vi "AlliGator Decay Fit Parameter Map Actions.vi"(0 "AlliGator Q Elements in":T6[](array[typedef]), 1 "VI in":refnum<vi>, 2 "Script in":bool, 5 "data value reference":refnum<data-value>, 7 "AlliGator Q Event in":T7=enum."GUI:Idle", 9 "Data":variant, 11 "error in (no error)":errorcluster, 12 "AlliGator Ctrl Refnums":T8) -> (3 "Script out":bool, 4 "AlliGator Q Elements out":T6[](array[typedef]), 6 "Data Value Reference out":refnum<data-value>, 10 "[Notebook Message]":T1[](array[typedef]) {"Message Style"."Font Size" min=6.0 step=1.0}, 15 "error out":errorcluster)   [LabVIEW 2021, in "AlliGator Decay Fit Parameter Map.lvlib"]
doc: "Processes AlliGator decay fit parameter map-related actions."
uses:
  AlliGator/Decay Fit Parameter Map/AlliGator Decay Fit Parameter Map.lvlib
  AlliGator/Internal Variables/AlliGator Internal Variables v2.ctl
  <vilib>/vision/Image Controls.llb/IMAQ Image.ctl
  AlliGator/Internal Variables/AlliGator Gate Image Set.ctl
  AlliGator/Files/AlliGator FLI Dataset Type.ctl
  AlliGator/Files/AlliGator Data Series Type.ctl
  AlliGator/Dual-Channel Datasets/AlliGator Dataset Channel.ctl
  AlliGator/Settings/AlliGator Gate Arithmetic.ctl
  AlliGator/Source Image/AlliGator Displayed Image.ctl
  Image/Named ROI Description.ctl
  AlliGator/Phasor Graph/AlliGator Decay Metadata v3.ctl
  AlliGator/Decay Analysis/Decay Preprocessing/AlliGator Decay Background Subtraction Info.ctl
  AlliGator/Decay Analysis/Decay Preprocessing/AlliGator Baseline Subtraction Method.ctl
  Graphs/XY Graph/XY Graph Plot Shift Parameters.ctl
  Graphs/XY Graph/XY Graph Plot Shift Method.ctl
  AlliGator/Decay Analysis/Decay Preprocessing/AlliGator Decay Extrapolation Parameters.ctl
  Phasor/Calibration Phasor (m, phi).ctl
  Phasor/Phasor Reference Series.ctl
  Phasor/Phasor Calibration Map v2.ctl
  Phasor/Phasor (g, s).ctl
  AlliGator/Phasor Graph/AlliGator Raw Phasor Plot Data v5.ctl
  Phasor/Phasor Standard Deviation Options.ctl
  AlliGator/Phasor Plot/AlliGator Phasor Multi-Harmonic Data.ctl
  Phasor/Phasor Harmonic Data.ctl
  AlliGator/Decay Fit Parameter Map/AlliGator Decay Fit Options & Parameters v4.ctl
  Fits/IRF(X)PSED/Decay Fit Options v4.ctl
  Fits/Decay Convolution/Decay Model.ctl
  Fits/Residual Type.ctl
  Fits/IRF(X)PSED/Fit Weights Type v2.ctl
  Fits/Non-linear Fitting Method v2.ctl
  Fits/Fit Calculation Method.ctl
  Fits/Non-linear Fitting Algorithm.ctl
  AlliGator/Decay Analysis/Decay Fit/AlliGator Decay Fit Parameter Constraints 2.ctl
  Fits/IRF(X)PSED/Decay Fit Parameters In List.ctl
  Fits/IRF(X)PSED/MLE Baseline Offset Type.ctl
  AlliGator/Decay Analysis/Decay Preprocessing/AlliGator Decay Preprocessing Parameters.ctl
  Fits/IRF(X)PSED/Decay Fit Parameters & Derived Quantities List v2.ctl
  Fits/IRF(X)PSED/Decay Fit Result Constraint.ctl
  AlliGator/Decay Fit Parameter Map/AlliGator Parameter Maps Data.ctl
  AlliGator/Action Engine/AlliGator Q Event.ctl
  AlliGator/GUI/AlliGator Ctrl Refnums.ctl
  AlliGator/GUI/AlliGator Other Ctrl Refnums.ctl
  AlliGator/GUI/AlliGator State Indicator.ctl
  AlliGator/GUI/AlliGator Main Window Tabs.ctl
  AlliGator/GUI/AlliGator Phasor Plot Ctrl Refnums.ctl
  AlliGator/GUI/AlliGator Phasor Graph Ctrl Refnums.ctl
  Phasor/Phasor Calibration Type.ctl
  AlliGator/GUI/AlliGator Dataset Ctrl Refnums.ctl
  AlliGator/GUI/AlliGator Registered Events Ctrl Refnums.ctl
  AlliGator/GUI/AlliGator Image Histogram Control Refnums.ctl
  Histograms/Linear Histogram Options.ctl
  Histograms/Histogram Bin Option.ctl
  Histograms/Histogram Bin Position.ctl
  AlliGator/Decay Fit Parameter Map/AlliGator Decay Fit Map Control Refnums.ctl
  AlliGator/Parameter Map/AlliGator Parameter Map Control Refnums.ctl
  AlliGator/Action Engine/AlliGator Q Element.ctl
  Notebook/Notebook Message Object.ctl
  Rich Text Box/Text Formatting.ctl
  Rich Text Box/Text Colors.ctl
  Rich Text Box/Text Style.ctl
  Rich Text Box/Text Alignment.ctl
  AlliGator/Action Engine/Alligator Elements Order in Action Stack.ctl
  AlliGator/Globals, Variables, Constants/AlliGator Variables List.ctl
  AlliGator/GUI/AlliGator Image Display Type.ctl
  Palette/Image Palette Information.ctl
  Image/Image Display Palette Type.ctl
  Files/Load-Save File Info.ctl
  Rich Text Box/Text Format List.ctl
  AlliGator/GUI/AlliGator Image Mouse Up Event Data.ctl
  Image/Image ROI Descriptor.ctl
  Image/Image Contour Definition.ctl
  Image/Image Contour ID.ctl
  Image/Image ROI Type.ctl
  Image/Image Control Refnum.ctl
  AlliGator/Decay Fit Parameter Map/AlliGator Decay Parameter Map Update Event Data.ctl
  AlliGator/GUI/AlliGator Windows List.ctl
  c5217346-0728-4db9-a30e-52dae72b7cfc.vi
  Variant/Variant to Data/Variant to Boolean.vi
  AlliGator/Action Engine/AlliGator Add Single Action to Stack.vi
  Variant/Variant to Data/Variant to [String].vi
  Variant/Variant to Data/Variant to String.vi
  Variant/Variant to Data/Variant to I32.vi
  AlliGator/Local Decay Window/AlliGator Local Decay Window.lvlib
  Fits/Fits.lvlib
  AlliGator/Action Engine/AlliGator Action Engine.lvlib
  GUI/GUI.lvlib
  Variant/Variant to Data/Variant to Data.lvlib
  AlliGator/Globals, Variables, Constants/AlliGator Globals, Variables & Constants.lvlib
  Palette/Palette.lvlib
  AlliGator/GUI/AlliGator GUI.lvlib
  Image/Image.lvlib
  Files/Files.lvlib
  Sound/Sound.lvlib
  AlliGator/Parameter Map/AlliGator Parameter Map.lvlib
  Utilities/Utilities.lvlib
  Notebook/Notebook.lvlib
  Phasor/Phasor.lvlib
  AlliGator/Decay Analysis/Decay Preprocessing/AlliGator Decay Preprocessing.lvlib
  Graphs/XY Graph/XY Graph Add-Ons.lvlib
  AlliGator/Phasor Graph/AlliGator Phasor Graph.lvlib
  AlliGator/Files/AlliGator Files.lvlib
  AlliGator/Internal Variables/AlliGator Internal Variables.lvlib
  AlliGator/Phasor Plot/AlliGator Phasor Plot.lvlib
  AlliGator/Source Image/AlliGator Source Image.lvlib
  AlliGator/Decay Analysis/Decay Fit/AlliGator Decay Fit.lvlib
  AlliGator/Settings/AlliGator Settings.lvlib
  Rich Text Box/Rich Text Box.lvlib
  AlliGator/Dual-Channel Datasets/AlliGator Dual-Channel Datasets.lvlib
  Histograms/Histogram Window.lvlib
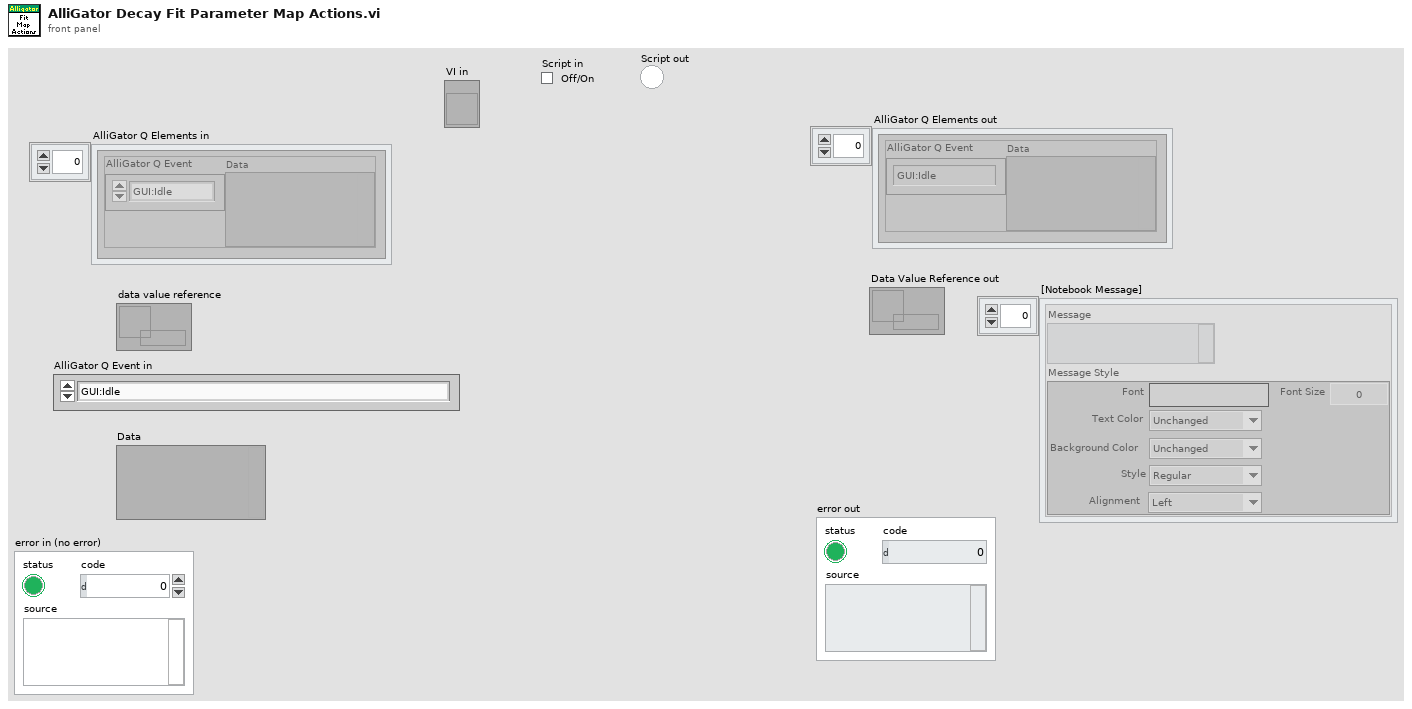
[diagram p1: front panel]
types:
  T1 = typedef "Notebook.lvlib/Notebook Message Object.ctl" = cluster{"Message":string, "Message Style":T2}
  T2 = typedef "Rich Text Box.lvlib/Text Formatting.ctl" = cluster{"Font":string, "Text Color":T3, "Background Color":T3, "Style":T4, "Font Size":dbl, "Alignment":T5}
  T3 = typedef "Rich Text Box.lvlib/Text Colors.ctl" = enum16{"Unchanged", "Black", "Blue", "Cyan", "Maroon", "Gray", "Violet", "Green", "Light Green", "Orange", "Yellow", "Magenta", "Red", "White"}
  T4 = typedef "Rich Text Box.lvlib/Text Style.ctl" = enum16{"Regular", "Bold", "Italic", "Underline", "Strikeout"}
  T5 = typedef "Rich Text Box.lvlib/Text Alignment.ctl" = enum16{"Left", "Right", "Center"}
  T6 = typedef "AlliGator Action Engine.lvlib/AlliGator Q Element.ctl" = cluster{"AlliGator Q Event":T7, "Data":variant}
  T7 = typedef "AlliGator Action Engine.lvlib/AlliGator Q Event.ctl" = enum16{"---- Files ----", "Files:Set Batch Export Files To Save", "Files:Set Dataset Loading & Pre-processing Options", "Files:Check #Frames in Dataset", "Files:Increment Frame Index", "Files:Open Mask Image", "Files:Open White Light Image", "Files:Open Single Dataset", "Files:New Folder of Folders Selected", "Files:Load File (all Types)_Scriptable", "Files:Move Flattened Series to Folders Series", "Files:Select Folder", "Files:Load FLI Dataset", "Files:Load Swiss SPAD 1 Dataset", "Files:Load Swiss SPAD 2 Dataset", "Files:Load .sdt FLI Dataset", "Files:Load .ptu FLI Dataset", "Files:Load .bin FLI Dataset", "Files:Load Single Gate Image Folder", "Files:Load I/m/phi Dataset (deprecated)", "Files:Load Single Image", "Files:Subtract Background File", "Files:Export FLI Dataset", "Files:Load HDF5 FLI Dataset", "Files:Set Destination File Path", "Files:Save Mask Image", "Files:Batch Conversion", "Files:New Folder Selected", "Files:Close FLI Dataset", "Files:Close FLI Dataset Series", "Files:Close White Light Image", "Files:Close Mask Image", "---- FLI Dataset ----", "FLI Dataset:Channel Arithmetic", "FLI Dataset:Export Average Lifetime Map as ASCII", "FLI Dataset:Export User-Defined Quantity Map as ASCII", "FLI Dataset:Python Function FLI Dataset Event", "FLI Dataset:ROI Analysis", "FLI Dataset:Tilted Logistic Square Gated IRF Characteristics Map", "FLI Dataset:Logistic Square Gated IRF Characteristics Map", "FLI Dataset:Square Gated IRF Characteristics Map", "FLI Dataset:Multi-ROI Single-Pixel Phasor Analysis", "FLI Dataset:Multi-ROI Single-Pixel NLSF Analysis", "FLI Dataset:All ROIs IRF Extraction", "FLI Dataset:All ROIs Decay Fit Non-Interactive (Fast + Individual IRF)", "FLI Dataset:All ROIs Phasor Analysis", "FLI Dataset:All ROIs Decay Fit", "FLI Dataset:Fluorescence Decay Statistics", "FLI Dataset:Update Decay Statistics Graph", "FLI Dataset:Get Decay from ROI", "FLI Dataset:All ROIs Average Lifetimes", "FLI Dataset:Save/Load Local IRFs", "FLI Dataset:Clear Local IRFs", "FLI Dataset:Phasor Calibration Maps (# Gates Series) Script", "FLI Dataset:Calibrated Phasor Map Series", "---- FLI Dataset Series ----", "FLI Dataset Series:Sum All Datasets in Series", "FLI Dataset Series:Add Dataset to Accumulated Dataset", "FLI Dataset Series:Display Accumulated Dataset", "FLI Dataset Series:Clear Dataset Series Sum", "FLI Dataset Series:Time-Series Analysis (NLSF)", "FLI Dataset Series:Time-Series Analysis (Phasor)", "---- Image ----", "Image:Update Image Profile Plots", "Image:Image Histogram Cursor Move", "Image:Image Histogram", "Image:Image Contrast", "Image:Set Image Histogram Cursor Move Flag", "Image:Clear Image Overlay", "Image:Use ROI as Search Area", "Image:Set ROI Diameter", "Image:Save Image Data as TIFF", "Image:Save Displayed Image with Overlay", "Image:Save Image Overlay Only", "Image:Save Image as Hot Pixel Mask", "Image:Change Source Image Color Palette", "Image:Copy Image to Clipboard", "Image:Source Image ROI Selection", "Image:Delete All ROIs", "Image:Delete All Unselected ROIs", "Image:Delete ROI", "Image:Merge All ROIs", "Image:Store ROI", "Image:Source Image ROI Storage", "Image:Export ROI Description to Notebook", "Image:Save ROI", "Image:Load ROI", "Image:Paste ROI Definition", "Image:Clear ROI", "Image:Identify ROIs in Mask Image", "Image:Create Complementary ROI", "Image:Create Contour ROI", "Image:Create ROI(s) from Pixels with Peak above Min_Scriptable", "Image:Create ROI(s) from Pixels with Intensity above Min_Scriptable", "Image:Compute ROI Statistics", "Image:Delete ROI(s) based on ROI Characteristics", "Image:Create ROI Grid", "Image:ROI to Individual Pixel ROIs", "Image:Python Function Source Image Event", "Image:Show Phasor Calibration Map ROI Centers", "Image:Convert ROI to Mask Image", "Image:Mouse Move", "Image:Mouse Up", "Image:Set Source Image Mouse Move Flag", "Image:Add Scale Bar Overlay", "Image:Delete Existing ROIs Option", "Image:Overlay ROI Median", "Image:Check Current ROI", "Image:Update True Pixel Value", "---- Decay ----", "Decay:Clear IRF/Reference Plot", "Decay:Add Decay to Graph", "Decay:Smoothen Plot", "Decay:Smoothen Plot Tail", "Decay:Average Selected Plots", "Decay:Extract IRF", "Decay:Optimal IRF Extraction", "Decay:Threshold IRF", "Decay:Fit to Model IRF", "Decay:Fit IRF to Square Gate", "Decay:Fit IRF to Logistic Square Gate", "Decay:Fit IRF to Tilted Logistic Square Gate", "Decay:Create Bounding Cursors Set", "Decay:Export Bounding Cursors Definition to Notebook", "Decay:Denoise Plot", "Decay:Compute Cumulative Function", "Decay:Use as Reference Decay", "Decay:Show Reference Decay/IRF", "Decay:Extrapolate Decay", "Decay:Create Head & Tail Bounding Cursors", "Decay:Store Cursor-defined Head & Tail Fractions", "Decay:Rebin Plot", "Decay:1-Normalize Decay", "Decay:[0-1]-Normalize Plot", "Decay:Straighten Decay", "Decay:Shift Decay", "Decay:Fold Decay", "Decay:Fit Decay", "Decay:Global Fit of Selected Decays", "Decay:Post Global Fit Script", "Decay:Add Global Fit Parameters to Graph", "Decay:Add Decay Parameter(s) to Plot (Graph)", "Decay:Export Decay to Phasor Graph", "Decay:Compute Average Lifetime", "Decay:Plot Convolution", "Decay:Graph Tip Strip Update", "---- Decay Statistics ----", "Decay Statistics:Tip Strip Update", "---- Intensity Time Trace ----", "Intensity Time Trace:Use File Timestamp", "Intensity Time Trace:Load Intensity Corrections File", "Intensity Time Trace:Clear Intensity Corrections File", "Intensity Time Trace:Tip Strip Update", "---- Phasor Plot ----", "Phasor Plot:Build Phasor Plot", "Phasor Plot:Change Phasor Plot Color Palette", "Phasor Plot:Adjust Phasor Plot Display Range", "Phasor Plot:Highlight Image ROI in Phasor Plot", "Phasor Plot:Save Phasor Plot Image with Overlay", "Phasor Plot:Export Complex Phasor Map", "Phasor Plot:Export Phasor Ratio Map", "Phasor Plot:Export Average Lifetime Map", "Phasor Plot:Compute Phase Lifetime Histogram", "Phasor Plot:Compute Phasor Ratio Histogram", "Phasor Plot:Compute Phase Lifetime vs Intensity Scatter Plot", "Phasor Plot:Weber 2-Component Decomposition", "Phasor Plot:Update Phasor Color Map Vertices", "Phasor Plot:Clear Phasor Overlay", "Phasor Plot:Use Segment Extremities as References", "Phasor Plot:Use UC/Segment Intersections as References", "Phasor Plot:Use UC/Principal Axis Intersections as References", "Phasor Plot:Use UC/Linear Fit Intersections as References", "Phasor Plot:Update Phasor Plot Reference", "Phasor Plot:Show Local Phasor Info in Phasor Plot", "Phasor Plot:Update Phasor Plot State", "Phasor Plot:Phasor Plot ROI Storage", "Phasor Plot:Phasor Plot ROI Selection", "Phasor Plot:Python Function Phasor Plot Event", "Phasor Plot:Overlay Phasor ROI, Ratio or Map in Source Image", "Phasor Plot:Compute Decay of Selected Phasors", "Phasor Plot:Phasor at Image Pixel", "Phasor Plot:Mouse Move", "Phasor Plot:Mouse Up", "Phasor Plot:Display Range Mouse Move", "Phasor Plot:Set Mouse Move Flag", "Phasor Plot:Update True Phasor Plot Value", "---- Phasor Graph ----", "Phasor Graph:Get Phasor Value", "Phasor Graph:Create New Phasor Plot Dialog", "Phasor Graph:Update Last Phasor Value", "Phasor Graph:Update Phasor (m, phi)", "Phasor Graph:Remove Single Phasor from Plot", "Phasor Graph:Add Single Phasor to Plot", "Phasor Graph:Remove Phasor Plot", "Phasor Graph:Remove Selected Phasor Plots", "Phasor Graph:Clear Phasor Data", "Phasor Graph:Clear Phasor Graph", "Phasor Graph:Cursor Move", "Phasor Graph:Draw Cursor Connecting Line", "Phasor Graph:Clear Cursor Connecting Line", "Phasor Graph:Find UC Intersection", "Phasor Graph:Use UC/Cursor-Defined Line Intersections", "Phasor Graph:Use Selected Plots Fitted Line/UC Intersections", "Phasor Graph:Use Selected Plots Principal Axis/UC Intersections", "Phasor Graph:Show Single Phasor", "Phasor Graph:Save Single Phasor Plot", "Phasor Graph:Save All Phasor Plots", "Phasor Graph:Load Phasor Plot(s)", "Phasor Graph:Phasor Multiplication", "Phasor Graph:Compute Average Phasor", "Phasor Graph:Compute Multiple Average Phasors (Selected Plots)", "Phasor Graph:Export Single Phasor Plot Phase Lifetimes", "Phasor Graph:Parameter 2 vs Parameter 1 Scatter Plot", "Phasor Graph:Use Cursor n Location", "Phasor Graph:Set Reference n to Current Phase Lifetime Value", "Phasor Graph:Set Reference n to Lifetime Value", "Phasor Graph:Set Cursor n Location", "Phasor Graph:Save Phasor Graph Image", "Phasor Graph:Update SEPL Plot", "Phasor Graph:Export Single Phasor Plot Data", "Phasor Graph:Export Selected Phasor Plots Data", "Phasor Graph:Python Function Phasor Graph Event", "Phasor Graph:Tip Strip Update", "---- Calibration ----", "Calibration:Set Calibration Type", "Calibration:Load/Save Phasor Calibration", "Calibration:Load/Save Phasor Calibration Series", "Calibration:Load/Save Phasor Calibration Map", "Calibration:Use as Calibration", "Calibration:Compute Optimal Calibration from Phasor References", "Calibration:Clear Phasor Calibration", "Calibration:Single Phasor Calibration Information", "Calibration:Use as Calibration Series", "Calibration:Use as Calibration Map", "Calibration:Clear Calibration Series", "Calibration:Phasor Calibration Series Information", "Calibration:Clear Calibration Map", "Calibration:Phasor Calibration Map Information", "Calibration:Apply Phasor Calibration", "Calibration:Update Single Plot Calibration", "Calibration:Update Multiple Plots Calibration", "Calibration:Clear Single Plot Calibration", "Calibration:Clear All Plots Calibrations", "Calibration:Clear Plot(s) Calibration(s)?", "---- Phasor Ratio ----", "Phasor Ratio:Clear Reference n", "Phasor Ratio:Toggle Selected Plot(s)  Lock to Reference 1", "Phasor Ratio:Use as Reference n", "Phasor Ratio:Send Reference n to Notebook", "Phasor Ratio:Toggle Selected Plot(s)  Lock to Reference 2", "Phasor Ratio:Compute Phasor Ratio at Mouse Location", "Phasor Ratio:Compute Phasor Plot's Average Phasor Ratio", "Phasor Ratio:Compute Time-Series Phasor Ratios", "Phasor Ratio:Fit Line to Phasor Ratio Plot", "Phasor Ratio:Save References", "Phasor Ratio:Load References", "Phasor Ratio:Update Phasor Reference 1", "Phasor Ratio:Update Phasor Reference 2", "Phasor Ratio:Move Cursor n to Reference n", "Phasor Ratio:Use as Phasor Reference 1 Lifetime", "Phasor Ratio:Use as Phasor Reference 2 Lifetime", "Phasor Ratio:Export Phasor Ratio Map as ASCII", "Phasor Ratio:Tip Strip Update", "---- Lifetime & Other Parameters Graph ----", "Lifetime:Compute Sliced Mean, SDV and CV Plots", "Lifetime:Plot Decay Shifts", "Lifetime:Plot Histogram", "---- Decay Fit Parameter Map ----", "Decay Fit Parameter Map:Export ROI NLSF Data as ASCII", "Decay Fit Parameter Map:Set Decay Fit Parameter Map Selection", "Decay Fit Parameter Map:Build Decay Fit Parameter Map", "Decay Fit Parameter Map:Change Decay Fit Parameter Map Color Palette", "Decay Fit Parameter Map:Export Decay Fit Parameter Map Data as ASCII", "Decay Fit Parameter Map:Export All Decay Fit Parameter Maps Data as ASCII", "Decay Fit Parameter Map:Selected Parameter Scatterplot", "Decay Fit Parameter Map:Parameter 2 vs Parameter 1 Scatterplot", "Decay Fit Parameter Map:Save Decay Fit Parameter Map Image", "Decay Fit Parameter Map:Save-Load IRFs & Fit Data", "Decay Fit Parameter Map:Update Local Decay Plots", "Decay Fit Parameter Map:Python Function Decay Fit Parameters Map Event", "Decay Fit Parameter Map:Overlay Decay Fit Parameter Map in Source Image", "Decay Fit Parameter Map:Selected Parameter vs Intensity Scatterplot", "Decay Fit Parameter Map:Mouse Up", "Decay Fit Parameter Map:Mouse Move", "Decay Fit Parameter Map:Display Range Mouse Move", "Decay Fit Parameter Map:Change Map Resolution", "Decay Fit Parameter Map:Variance Significance Maps", "Decay Fit Parameter Map:Fit Result Constraints Window", "---- Parameter Map ----", "Parameter Map:Export ROI Parameters Data as ASCII", "Parameter Map:Delete Parameter Map Set", "Parameter Map:Update Parameter List", "Parameter Map:Build Parameter Map", "Parameter Map:Change Parameter Map Color Palette", "Parameter Map:Export Parameter Map Data as ASCII", "Parameter Map:Export All Parameter Maps Data as ASCII", "Parameter Map:Selected Parameter Scatterplot", "Parameter Map:Parameter 2 vs Parameter 1 Scatterplot", "Parameter Map:Selected Parameter vs Intensity Scatterplot", "Parameter Map:Save Parameter Map Image", "Parameter Map:Save-Load IRFs & Parameter Maps (TODO)", "Parameter Map:Set Parameter Map Selection", "Parameter Map:Python Function Parameter Map Event", "Parameter Map:Overlay Parameter Map in Source Image", "Parameter Map:Update Local Decay Plots", "Parameter Map:Mouse Up", "Parameter Map:Mouse Move", "Parameter Map:Display Range Mouse Move", "---- Generic Graph ----", "Generic Graph:Generic XY Graph Event", "Generic Graph:Python Function XY Graph Event", "Generic Graph:New Plot", "Generic Graph:Save Plot", "Generic Graph:XY Plot Histogram", "Generic Graph:Set XY Graph Plot Name", "Generic Graph:Set Last Cursor Style", "Generic Graph:Tip Strip Update", "---- GUI ----", "GUI:Start Script", "GUI:Type of Displayed Image Changed", "GUI:Gate Image Slide Changed", "GUI:Show Busy Icon", "GUI:Show Busy Icon & Abort Button", "GUI:Hide Busy Icon", "GUI:Hide Busy Icon & Abort Button", "GUI:Abort", "GUI:End Script", "GUI:Start Timing", "GUI:End Timing", "GUI:Set State Indicator", "GUI:Send Parameters JSON Strings to Clipboard", "GUI:Set Gate Step", "GUI:Idle", "GUI:Initialization", "GUI:Quit", "GUI:Increment Dataset Index", "GUI:Set Dataset Index to -1", "GUI:Time Series Slider Moved", "GUI:Time Series Slider Changed", "GUI:Toggle Playback or Loop", "GUI:Playback Script", "GUI:Set Phasor Frequency", "GUI:Open Window", "GUI:Start Test Script", "GUI:End Test Script", "GUI:Set Verbose Mode", "GUI:Set Verbose Settings Mode", "DEBUG"}
  T8 = typedef "AlliGator GUI.lvlib/AlliGator Ctrl Refnums.ctl" = cluster{"Other AlliGator Ctrl Refnums":T9, "Phasor Plot Ctrl Refnums":T10, "Phasor Graph Ctrl Refnums":T11, "Dataset Control Refnums":T12, "Registered Events Ctrl Refnums":T13, "Image Histogram Ctrl Refnums":T14, "Decay Fit Map Ctrl Refnums":T15, "Parameter Map Ctrl Refnums":T16}
  T9 = typedef "AlliGator GUI.lvlib/AlliGator Other Ctrl Refnums.ctl" = cluster{"State Indicators":refnum<vi>, " Progress Bar":refnum<vi>, "Decay Graph Active":refnum<vi>, "Decay Statistics Bin":refnum<vi>, "Time Step":refnum<vi>, "Use File Timestamp":refnum<vi>, "Tab Control":refnum<vi>, "CPU":refnum<vi>, "Abort Fit":refnum<vi>, "Dataset File/Folder Path":refnum<vi>, "Abort ROI Creation":refnum<vi>, "Event LED":refnum<vi>, "Dataset File/Folder Path 2":refnum<vi>, "Dataset File/Folder Path 3":refnum<vi>, "Dataset File/Folder Path 4":refnum<vi>, "Dataset File/Folder Path 5":refnum<vi>, "Dataset File/Folder Path 6":refnum<vi>, "Dataset File/Folder Path 7":refnum<vi>, "Dataset File/Folder Path 8":refnum<vi>, "Dataset File/Folder Path 9":refnum<vi>, "Dataset File/Folder Path 10":refnum<vi>, "Dataset File/Folder Path 11":refnum<vi>}
  T10 = typedef "AlliGator GUI.lvlib/AlliGator Phasor Plot Ctrl Refnums.ctl" = cluster{"Phasor Ratio":refnum<vi>, "Modulus Lifetime":refnum<vi>, "Phasor at cursor (m, phi)":refnum<vi>, "Phase Lifetime":refnum<vi>, "Phasor at cursor (g, s)":refnum<vi>, "Phasor Plor Average Lifetime":refnum<vi>, "Phasor Plot Active":refnum<vi>, "Save Phasor Plot":refnum<vi>, "Image Overlay Color":refnum<vi>, "Phasor Plot Color Scale":refnum<vi>, "Reference 1 Button":refnum<vi>, "Reference 2 Button":refnum<vi>, "True Phasor Plot Value":refnum<vi>}
  T11 = typedef "AlliGator GUI.lvlib/AlliGator Phasor Graph Ctrl Refnums.ctl" = cluster{"Phasor Ratio":refnum<vi>, "Modulus Lifetime":refnum<vi>, "Phasor at cursor (m, phi)":refnum<vi>, "Phase Lifetime":refnum<vi>, "Phasor at cursor (g, s)":refnum<vi>, "Phasor Graph Average Lifetime":refnum<vi>, "Phasor Graph Active":refnum<vi>, "Save Phasor Graph":refnum<vi>, "Phasor Frame Slide":refnum<vi>, "Single Step Phasor":refnum<vi>, "Calibration Type":refnum<vi>, "Show Line":refnum<vi>, "Phase Lifetime 1":refnum<vi>, "Phase Lifetime 2":refnum<vi>, "Phasor Graph Frequency":refnum<vi>, "Phasor Reference 1 Control":refnum<vi>, "Phasor Reference 2 Control":refnum<vi>, "Calibration Lifetime":refnum<vi>, "Phase Lifetime SDV":refnum<vi>, "Average Lifetime SDV":refnum<vi>, "Phasor Ratio SDV":refnum<vi>, "Modulus Lifetime SDV":refnum<vi>}
  T12 = typedef "AlliGator GUI.lvlib/AlliGator Dataset Ctrl Refnums.ctl" = cluster{"Current Data":refnum<vi>, "Gate Image Slide":refnum<vi>, "Time Point Slide":refnum<vi>, "Current Time Stamp":refnum<vi>, "Save Image":refnum<vi>, "Displayed Image":refnum<vi>, "Overlay Mode":refnum<vi>, "Phasor Overlay Color":refnum<vi>, "Image Color Scale":refnum<vi>, "Use ROI as Search Area":refnum<vi>, "Source Image ROI Color":refnum<vi>, "True Pixel Value":refnum<vi>}
  T13 = typedef "AlliGator GUI.lvlib/AlliGator Registered Events Ctrl Refnums.ctl" = cluster{"Time Point Slider":refnum<vi>, "Phasor Plot Display Range":refnum<vi>, "Decay Graph":refnum<vi>, "Decay Statistics Graph":refnum<vi>, "Intensity Time Trace":refnum<vi>, "Phasor Graph":refnum<vi>, "Phasor Ratio Graph":refnum<vi>, "Lifetime Graph":refnum<vi>, "Phasor Plot Display":refnum<vi>, "Source Image Display":refnum<vi>, "Decay Fit Parameter Map Display Range":refnum<vi>, "Decay Fit Parameter Map Display":refnum<vi>, "Parameter Map Display Range":refnum<vi>, "Parameter Map Display":refnum<vi>, "Phasor Plot Display Range":refnum<vi>}
  T14 = typedef "AlliGator GUI.lvlib/AlliGator Image Histogram Control Refnums.ctl" = cluster{"Image Histogram":refnum<vi>, "Image Histogram Options":refnum<vi>, "Image Histogram Active":refnum<vi>, "Image Histogram Upper Percentile":refnum<vi>, "Image Histogram Lower Percentile":refnum<vi>, "Auto-Adjust Contrast":refnum<vi>}
  T15 = typedef "AlliGator Decay Fit Parameter Map.lvlib/AlliGator Decay Fit Map Control Refnums.ctl" = cluster{"Decay Fit Parameter Map Color Scale":refnum<vi>, "Decay Fit Parameter":refnum<vi>, "Max Parameter":refnum<vi>, "Min Parameter":refnum<vi>, "Decay Fit Parameter Map Display":refnum<vi>, "Decay Fit Parameter Map Display Range":refnum<vi>, "Decay Parameter Map X":refnum<vi>, "Decay Parameter Map Y":refnum<vi>, "Decay Parameter Map Value":refnum<vi>}
  T16 = typedef "AlliGator Parameter Map.lvlib/AlliGator Parameter Map Control Refnums.ctl" = cluster{"Parameter Map Color Scale":refnum<vi>, "Map Parameter":refnum<vi>, "Max Parameter":refnum<vi>, "Min Parameter":refnum<vi>, "Parameter Map Display":refnum<vi>, "Parameter Map Display Range":refnum<vi>, "Parameter Map Set":refnum<vi>, "Parameter Map X":refnum<vi>, "Parameter Map Y":refnum<vi>, "Parameter Map Value":refnum<vi>}
  T17 = typedef "AlliGator Action Engine.lvlib/Alligator Elements Order in Action Stack.ctl" = enum16{"Enqueue 2 AFTER 1", "Enqueue 2 BEFORE 1"}
  T18 = typedef "AlliGator GUI.lvlib/AlliGator Image Display Type.ctl" = enum16{"Source Image", "Phasor Plot", "Decay Fit Parameter Map", "Parameter Map"}
  T19 = typedef "AlliGator Globals, Variables & Constants.lvlib/AlliGator Variables List.ctl" = enum16{"---- GUI ----", "GUI:Initialization Status", "GUI:State Indicators Refnum", "GUI:Original AlliGator Menu Items", "GUI:Current Action Loop State", "GUI:Script in progress", "GUI:Playback", "GUI:Loop Playback", "GUI:Search ROI Used", "GUI:Search ROI", "Decay Graph Max Legend Size", "Intensity Graph Max Legend Size", "Decay Statistics Graph Max Legend Size", "Phasor Graph Max Legend Size", "Phasor Ratio Graph Max Legend Size", "Lifetime Graph Max Legend Size", "---- Files ----", "Files:Export Dataset Frames as Individual Files", "Files:Show Batch Export Help Balloons", "Files:Frames in Dataset", "Files:ptu File Frame Start Indices", "Files:Current Frame in Dataset", "Files:Current Frame Timestamp", "Files:Dataset Loaded", "Files:Dataset Metadata", "Files:Dataset Channel", "Files:Dataset Data Description", "Files:Background Dataset Metadata", "Files:Background Dataset Channel", "Files:Background Dataset Data Description", "Files:Background File Subtraction", "Files:Background File Path", "Files:Background File Pile-up Correction", "Files:Background File Pixel Well Capacity", "Files:Background File Scaling Factor", "Files:Current Dataset Load Settings", "Files:Dataset Path", "Files:ICCD-specific Information", "Files:Macrotime Gate Separation", "------ Python Plugins ------", "Python Plugins:Information", "Python Plugins:Python Session", "Python Plugins:Valid Python Session?", "---- Source Image ----", "Source Image:ROIs", "Source Image:Current ROI", "Source Image:ROI Event Refnum", "X_Source Image:Display Range", "X_Source Image:Palette Information", "X_Source Image:Type of Displayed Image", "X_Time Gate Slider", "Source Image:Palette List", "Source Image:Scale", "Source Image:ROI Overlay Color", "Source Image:Overlay to Erase", "Source Image:Is Displayed Image Accumulated", "Source Image:White Light Image Modified", "Source Image:Mask Image Modified", "---- Image Profile Window ----", "Image Profile:Window Event Refnum", "Image Profile:IntensityType", "Image Profile:Intensity Average Type", "Image Profile:Intensity-weighted SDV", "Image Profile:Box Profile Type", "Image Profile:Window Open", "Image Profile:Plotted Fit Parameter", "------ Phasor Graph -------", "Phasor Graph:Show Line", "---- Phasor Plot ---", "Phasor Plot:Parameters Changed", "Phasor Plot:FLI Dataset Modified since last Calculation", "Phasor Harmonics Data", "Selected Phasor Harmonics", "Phasor Harmonic Manager Event Refnum", "Phasor Plot:ROIs", "Phasor Plot:Current ROI", "Phasor Plot:ROI Event Refnum", "Phasor Plot:Image Reference Points", "Phasor Plot:Computed", "Phasor Plot:Palette Information", "Phasor Plot:Palette List", "Phasor Plot:Phasor Ratio Palette Information", "Phasor Plot:Phasor Ratio Palette List", "Phasor Plot:Image Scale", "Phasor Plot:Image Overlay to Erase", "Phasor Plot:Image Elements to Update", "Phasor Plot:Current Calculation Parameters", "Phasor Plot:Current Calibration Options", "Phasor Plot:Reset Cumulated Phasor Plot", "Phasor Plot:Reference 1", "Phasor Plot:Lifetime Reference 1", "Phasor Plot:Reference 1 Frequency", "Phasor Plot:Reference 2", "Phasor Plot:Lifetime Reference 2", "Phasor Plot:Reference 2 Frequency", "---- Decay Analysis ----", "Number of Selected Decays to Fit", "LS Fit Results", "LAR Fit Results", "BS Fit Results", "Last Decay Max - Min", "Best Fit Parameters", "Best Fit Parameter Names", "Actual Size X", "Actual Size Y", "Binning X", "Binning Y", "Actual # Gates", "Dataset Number", "Gates to...", "Gates Skipped", "Gates to keep", "Gate Step", "Gate Separation", "Reversed Gates", "Pile-up Correction", "Pixel Well Capacity", "Background Subtracted", "Background Subtraction Method", "Background Definition Range", "Background File (deprecated)", "Number of Dataset Accumulated", "Array of Accumulated Dataset Paths", "Do Averaged Datasets", "Destination File Path", "Process Plot Target", "Use 1/D as Phasor Frequency", "---- Decay Fit Parameter Map -----", "Decay Fit Parameter Map:Palette Information", "Decay Fit Parameter Map:Palette List", "Decay Fit Parameter Map:X Resolution", "Decay Fit Parameter Map:Y Resolution", "Decay Fit Parameter Map:Use Decay Fit Result Constraints", "Decay Fit Parameter Map:Decay Fit Result Constraints", "Decay Fit Parameter Map:Decay Fit Result Constraints Applied", "---- Parameter Map ----", "Parameter Map:Palette Information", "Parameter Map:Palette List", "------- Local Decay Window ---------", "Local Decay Graph Window:Event Refnum", "Local Decay Graph Window:Use normalized IRF for convolution", "----- Miscellaneous ----", "Misc:Skippable Dialog Windows Status"}
  T20 = typedef "Palette.lvlib/Image Palette Information.ctl" = cluster{"Palette Name [# Colors,int?,inv?]":string, "Palette Type":T21, "Palette Colors":u32[], "Interpolate?":bool}
  T21 = typedef "Image.lvlib/Image Display Palette Type.ctl" = u32
  T22 = typedef "Files.lvlib/Load-Save File Info.ctl" = cluster{"Load/Save":bool, "File Path":path}
  T23 = typedef "Notebook.lvlib/Text Format List.ctl" = enum16{"Message", "Result", "Error", "Setting", "Verbose", "Warning"}
  T24 = typedef "Fits.lvlib/Decay Fit Parameters & Derived Quantities List v2.ctl" = enum16{"Offset", "Baseline", "A_1", "tau_1", "A_2", "tau_2", "<tau>_a", "f1_a", "f2_a", "<tau>_i", "f1_i", "f2_i", "-", "R^2", "Chi^2"}
  T25 = cluster{"Fit Parameter 1":T24, "Fit Parameter 2":T24}
  T26 = typedef "AlliGator GUI.lvlib/AlliGator Image Mouse Up Event Data.ctl" = cluster{"Current ROI Tool":u32, "ROI Descriptor":T27, "Shift":bool, "Alt":bool, "Image Display Refnum":T31}
  T27 = typedef "Image.lvlib/Image ROI Descriptor.ctl" = cluster{"Global Rectangle":i32[], "Contours":T28[]}
  T28 = typedef "Image.lvlib/Image Contour Definition.ctl" = cluster{"Contour Type":T29, "ROI Type":T30, "Points":i32[]}
  T29 = typedef "Image.lvlib/Image Contour ID.ctl" = enum32{"External", "Internal"}
  T30 = typedef "Image.lvlib/Image ROI Type.ctl" = enum16{"No Selection", "Point", "Line", "Rectangle", "Oval", "Polygon", "Freehand Region", "Annulus", "Unused2", "Unused3", "Broken Line", "Freehand Line", "Rotated Rectangle"}
  T31 = typedef "Image.lvlib/Image Control Refnum.ctl" = refnum<vi>
  T32 = typedef "AlliGator Decay Fit Parameter Map.lvlib/AlliGator Decay Parameter Map Update Event Data.ctl" = cluster{"Parameter":T24, "Parameter changed":bool}
  T33 = typedef "AlliGator GUI.lvlib/AlliGator Windows List.ctl" = enum16{"AlliGator Window", "Settings Window", "Notebook Window", "Dataset Information Window", "Source Image ROI Manager Window", "Phasor Plot ROI Manager Window", "Phasor Harmonic Manager Window", "Histogram Window", "Image Profile Window", "Local Decay Window", "About Window", "Batch Conversion Window", "Shot Noise Influence on Average Lifetime", "Fit Method Benchmark", "Camera Noise Influence on Lifetime", "AlliGator Alias Definition", "Fit Result Constraints Window"}
  T34 = typedef "Fits.lvlib/Decay Fit Parameters & Derived Quantities List.ctl" = enum16{"Offset", "Baseline", "A_1", "tau_1", "A_2", "tau_2", "<tau>_a", "f1_a", "f2_a", "<tau>_i", "f1_i", "f2_i", "-", "R^2", "Chi^2"}
  T35 = typedef "ROI Descriptor" = cluster{"Global Rectangle":i32[], "Contours":cluster{"ID":enum32{"External", "Internal"}, "Type":u32, "Coordinates":i32[]}[]}
  T36 = typedef "AlliGator Decay Fit Parameter Map.lvlib/AlliGator Power Law Parameters.ctl" = cluster{"Prefactor":dbl, "Exponent":dbl, "Offset":dbl}
  T37 = typedef "AlliGator Parameter Map.lvlib/AlliGator Parameter Map Update Event Data.ctl" = cluster{"Parameter":u16, "Parameter changed":bool, "Map Set":u16}
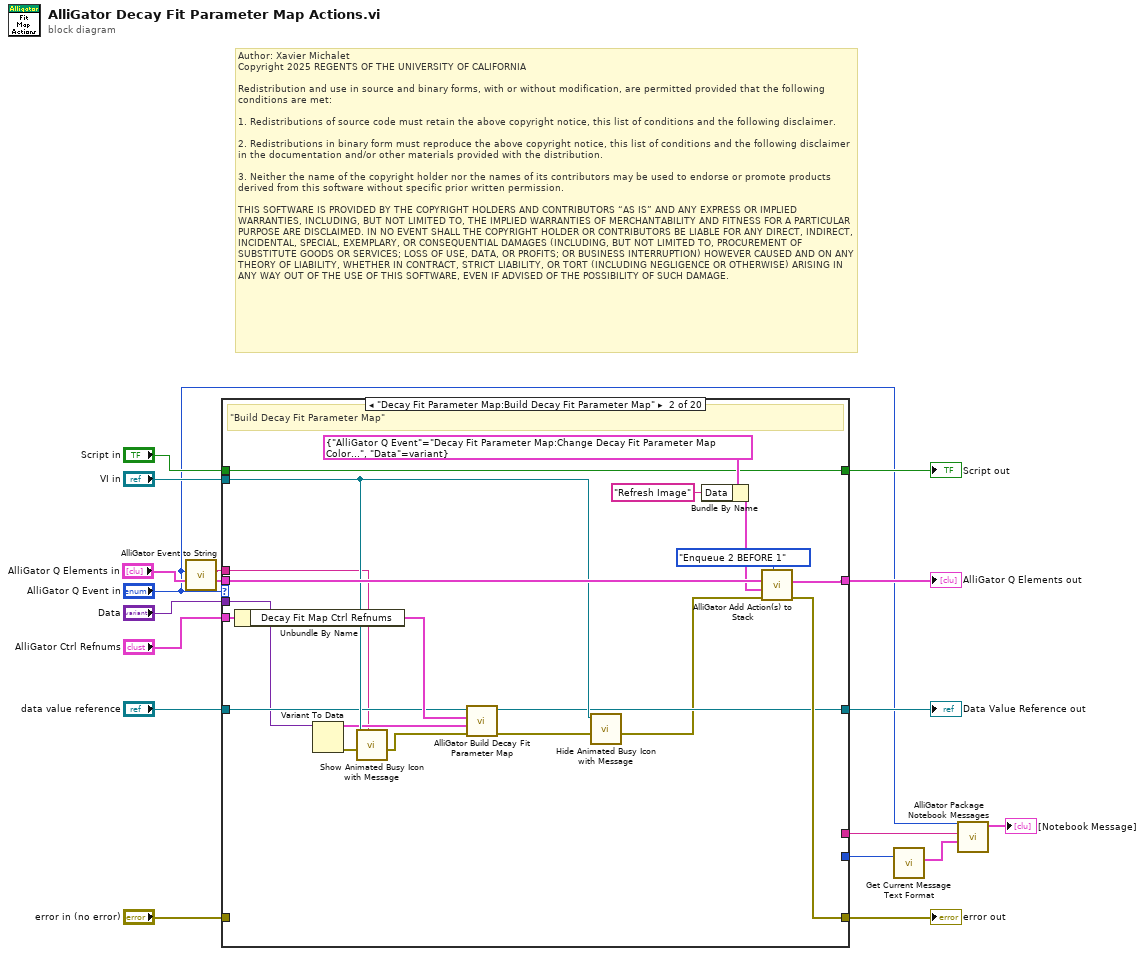
[diagram p0: block diagram]
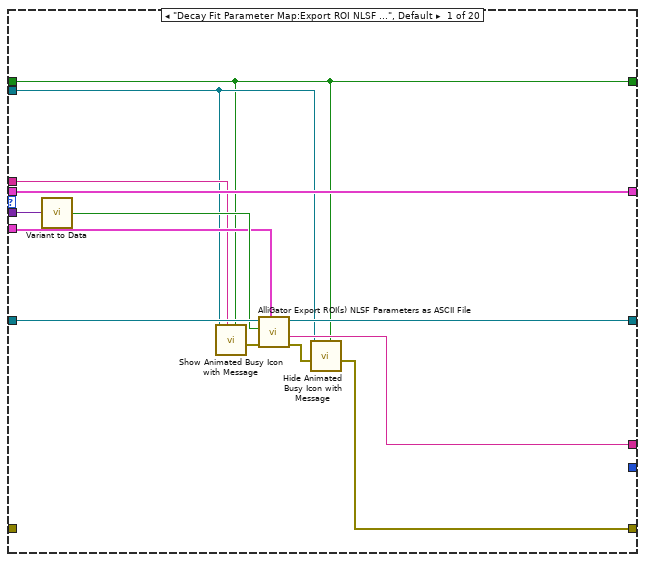
[diagram p2: hidden frame]
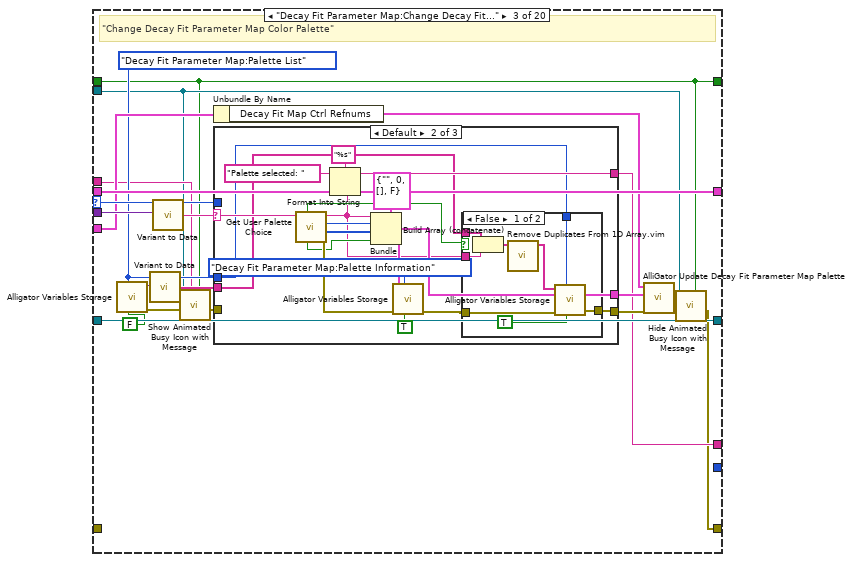
[diagram p3: hidden frame]
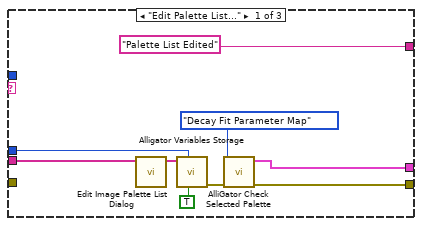
[diagram p4: hidden frame]
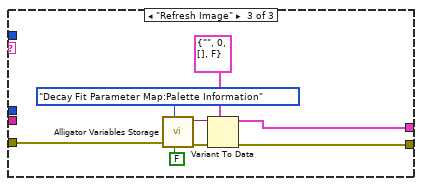
[diagram p6: hidden frame]
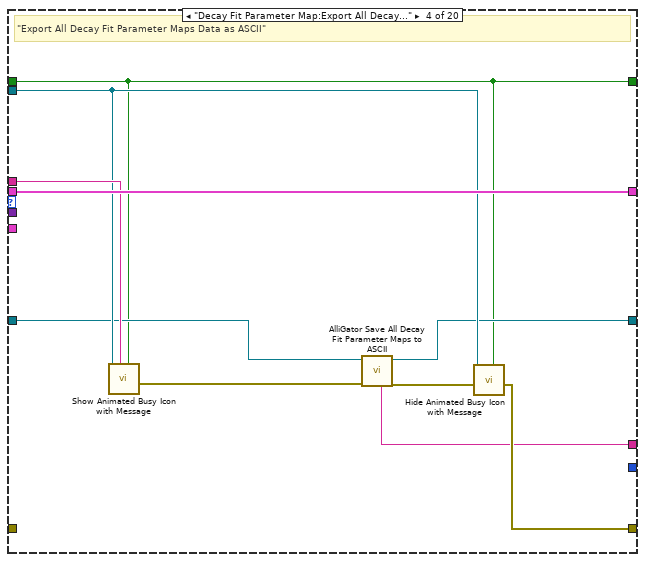
[diagram p7: hidden frame]
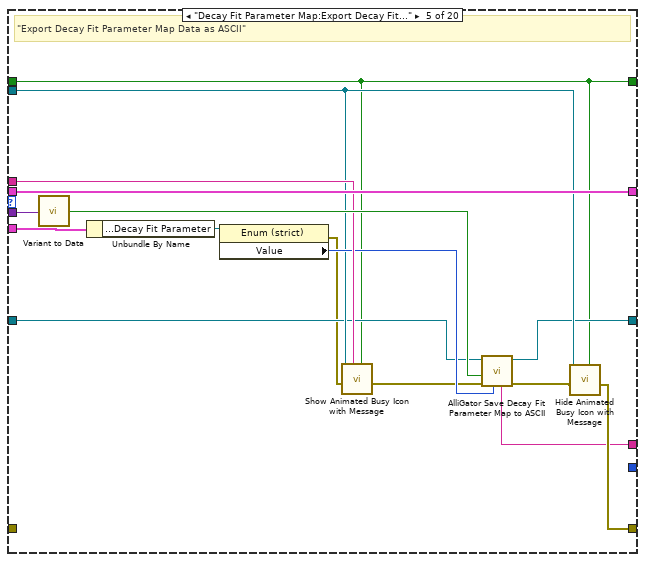
[diagram p8: hidden frame]
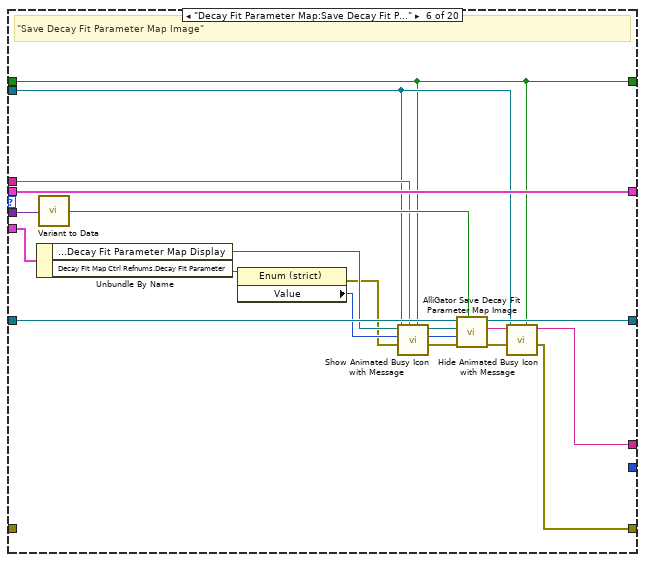
[diagram p9: hidden frame]
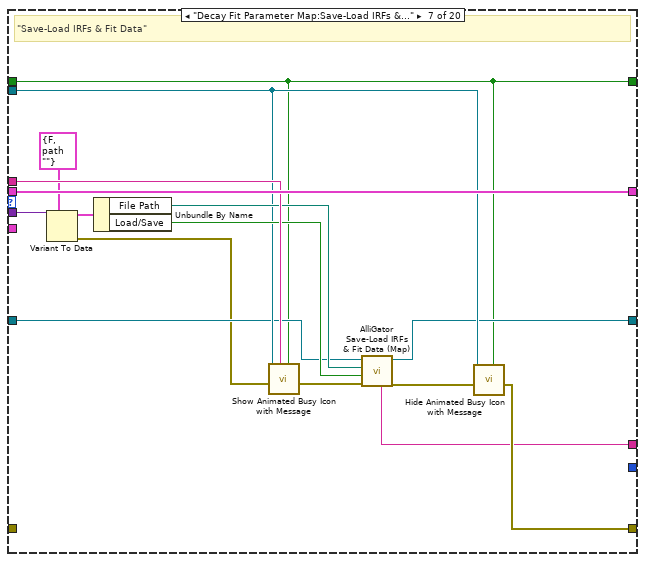
[diagram p10: hidden frame]
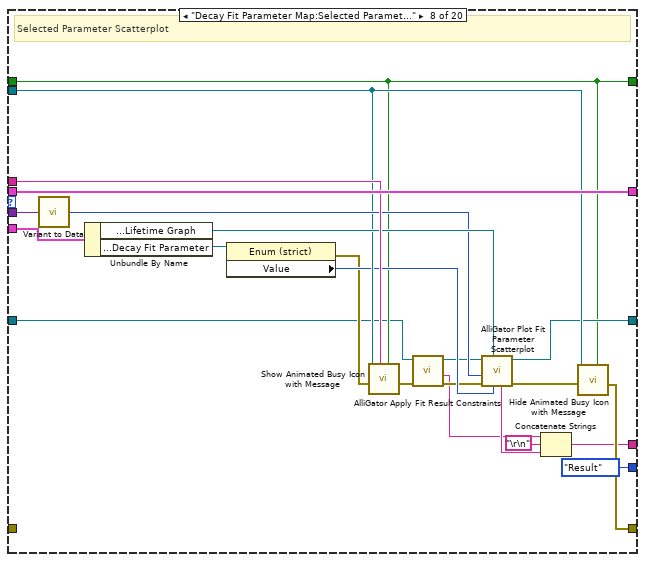
[diagram p11: hidden frame]
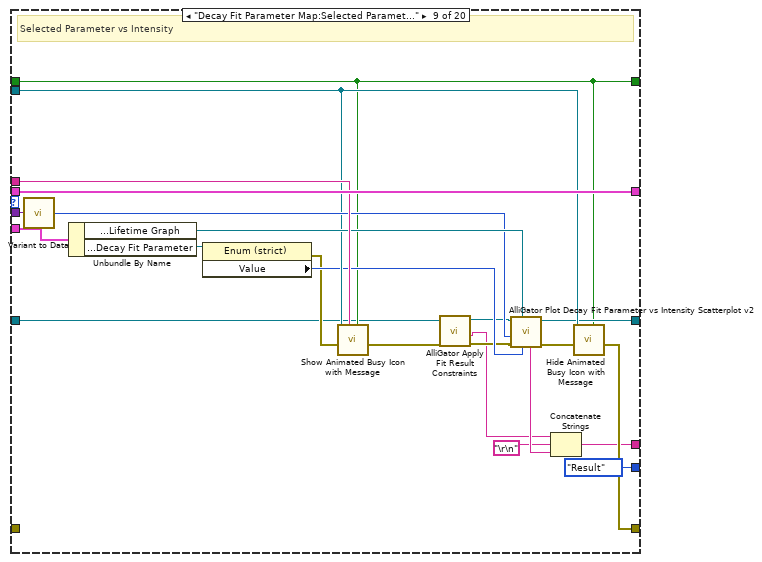
[diagram p12: hidden frame]
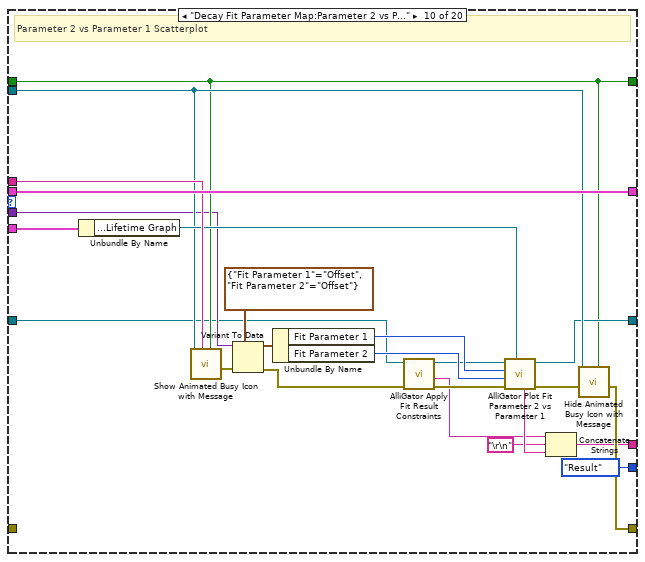
[diagram p13: hidden frame]
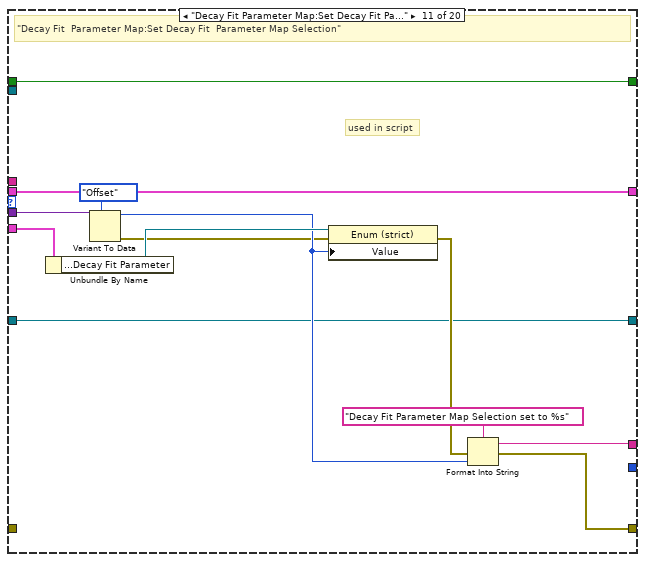
[diagram p14: hidden frame]
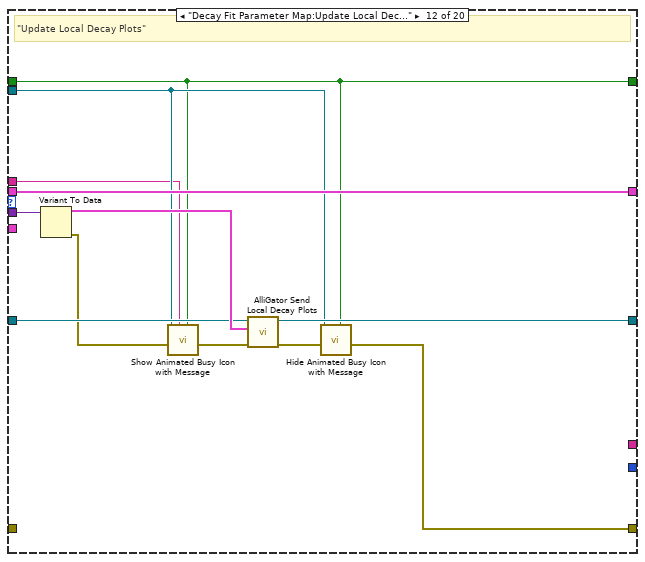
[diagram p15: hidden frame]
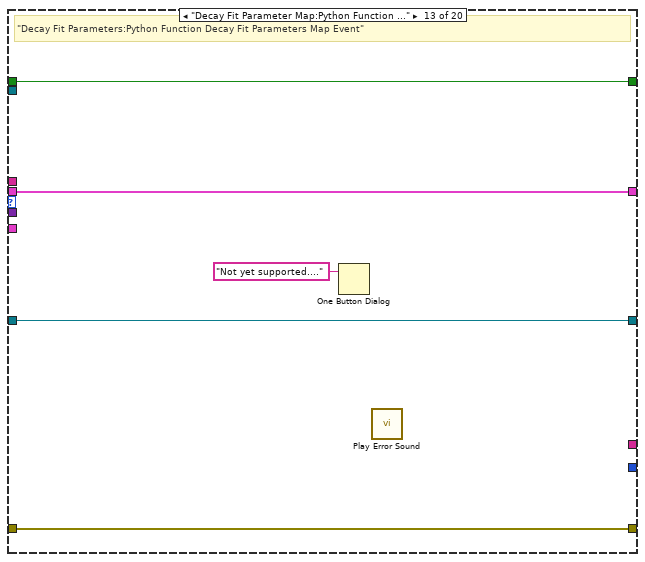
[diagram p16: hidden frame]
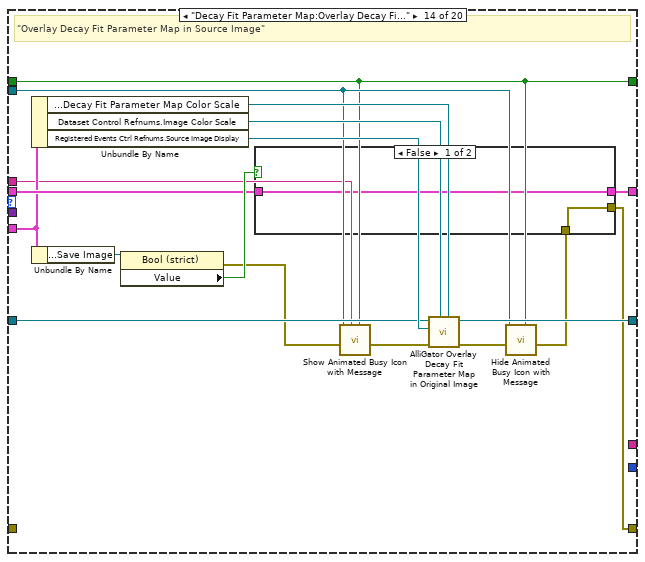
[diagram p17: hidden frame]
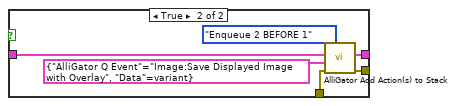
[diagram p18: hidden frame]
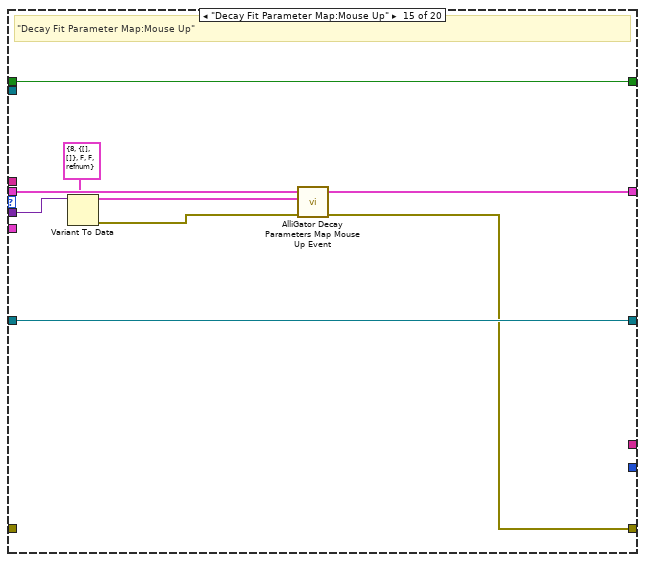
[diagram p19: hidden frame]
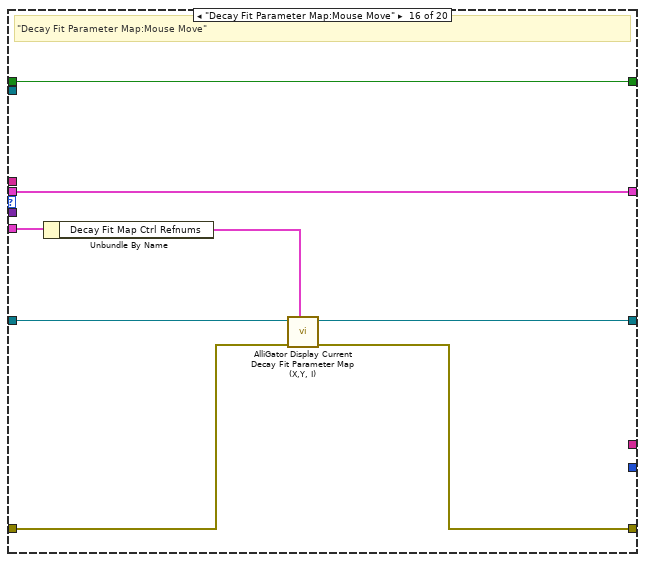
[diagram p20: hidden frame]
diagram:
  # "Author: Xavier Michalet\nCopyright 2025 REGENTS OF THE UNIVERSITY OF CALIFORNIA\n\nRedistribution and use in source and binary forms, with or without modification, are permitted provided that the following conditions are met:\n\n1. Redistributions of source code must retain the above copyright notice, this list of conditions and the following disclaimer.\n\n2. Redistributions in binary form must reproduce the above copyright notice, this list of conditions and the following disclaimer in the documentation and/or other materials provided with the distribution.\n\n3. Neither the name of the copyright holder nor the names of its contributors may be used to endorse or promote products derived from this software without specific prior written permission.\n\nTHIS SOFTWARE IS PROVIDED BY THE COPYRIGHT HOLDERS AND CONTRIBUTORS “AS IS” AND ANY EXPRESS OR IMPLIED WARRANTIES, INCLUDING, BUT NOT LIMITED TO, THE IMPLIED WARRANTIES OF MERCHANTABILITY AND FITNESS FOR A PARTICULAR PURPOSE ARE DISCLAIMED. IN NO EVENT SHALL THE COPYRIGHT HOLDER OR CONTRIBUTORS BE LIABLE FOR ANY DIRECT, INDIRECT, INCIDENTAL, SPECIAL, EXEMPLARY, OR CONSEQUENTIAL DAMAGES (INCLUDING, BUT NOT LIMITED TO, PROCUREMENT OF SUBSTITUTE GOODS OR SERVICES; LOSS OF USE, DATA, OR PROFITS; OR BUSINESS INTERRUPTION) HOWEVER CAUSED AND ON ANY THEORY OF LIABILITY, WHETHER IN CONTRACT, STRICT LIABILITY, OR TORT (INCLUDING NEGLIGENCE OR OTHERWISE) ARISING IN ANY WAY OUT OF THE USE OF THIS SOFTWARE, EVEN IF ADVISED OF THE POSSIBILITY OF SUCH DAMAGE."
  n1 = call "AlliGator Event to String.vi"("AlliGator Q Event"="AlliGator Q Event in") -> ("String"=w7:string)  [unwired: 8 in]
  n2 = case shown="\"Decay Fit Parameter Map:Build Decay Fit Parameter Map\"" "AlliGator Q Event in" {
    selector: "AlliGator Q Event in" -> [_ _ w70 _ _ _ _ _ _ _ _ _ _ _ _ _ _ _ _ _]
    tunnel: "Data" -> [w29 w34 w71 _ w140 w157 w171 w192 w215 w235 w256 w268 _ _ w304 _ w324 _ _ _]
    tunnel: "AlliGator Q Elements in" -> [w30 w50 w67 w125 w141 w158 w174 w197 w220 w244 w257 w269 w274 w283 w307 w317 w327 w353 w382 w395]
    tunnel: [w30 w49 w67 w125 w141 w158 w174 w197 w220 w244 w257 w269 w274 w282 w306 w317 w326 w352 w381 w395] -> w9
    tunnel: "VI in" -> [w19 w40 w52 w122 w133 w143 w166 w190 w213 w239 _ w260 _ w280 _ _ _ _ w377 _]
    tunnel: "Script in" -> [w18 w31 w51 w117 w128 w142 w161 w185 w208 w236 w245 w259 w270 w279 w308 w316 w328 w362 w376 w392]
    tunnel: w7 -> [w21 w32 w54 w123 w137 w145 w172 w195 w218 w242 _ w258 _ w278 _ _ _ _ w379 _]
    tunnel: "error in (no error)" -> [_ _ _ _ _ _ _ _ _ _ _ _ w273 _ _ w313 w321 w354 w386 w394]
    tunnel: [w20 w43 w53 w124 w138 w144 w173 w196 w219 w243 w246 w261 w273 w275 w305 w314 w325 w341 w378 w394] -> w14
    tunnel: "AlliGator Ctrl Refnums" -> [w25 w42 w66 _ w135 w156 _ w193 w216 w240 w253 _ _ w281 _ w315 w319 w345 w373 _]
    tunnel: "data value reference" -> [w28 w38 w63 w120 w131 w154 w164 w181 w205 w226 w248 w266 w272 w285 w309 w312 w329 w363 w387 w393]
    tunnel: [w27 w37 w63 w121 w132 w153 w165 w187 w210 w238 w248 w265 w272 w284 w309 w311 w329 w363 w368 w393] -> w17
    tunnel: [w23 _ w61 w116 w127 w152 w160 w178 w201 w224 w247 _ _ _ _ _ _ w339 w371 _] -> w4
    tunnel: [w18 w31 w51 w117 w128 w142 w161 w185 w208 w236 w245 w259 w270 w279 w308 w316 w328 w362 w376 w392] -> w6
    tunnel: [_ _ _ _ _ _ _ Text_Format_List."Result" ("Text Format") Text_Format_List."Result" ("Text Format") Text_Format_List."Result" ("Text Format") _ _ _ _ _ _ _ Text_Format_List."Result" ("Text Format") Text_Format_List."Result" ("Text Format") _] -> w1
    frame "Decay Fit Parameter Map:Export ROI NLSF Data as ASCII", Default {
      n3 = call-poly "Variant to Data.vi"("Variant"=w29) -> ("Value"=w26:bool)  [unwired: 8 in]
      n4 = call "Show Animated Busy Icon with Message.vi"("Already active? (F)"=w18, "Message"=w21, "Target VI Refnum"=w19) -> ("Error Out"=w22:errorcluster)  [unwired: 8 in]
      n5 = call "AlliGator Export ROI(s) NLSF Parameters as ASCII File.vi"("AlliGator Ctrl Refnums"=w25, "error in (no error)"=w22, "All ROIs"=w26, "AlliGator IV DVR in"=w28) -> ("error out"=w24:errorcluster, "Message"=w23:string, "AlliGator IV DVR out"=w27:refnum<data-value>)  [unwired: 5 in]
      n6 = call "Hide Animated Busy Icon with Message.vi"("Already active? (F)"=w18, "Error In"=w24, "Target VI reference"=w19) -> ("Error Out"=w20:errorcluster)  [unwired: 8 in]
    }
    frame "Decay Fit Parameter Map:Build Decay Fit Parameter Map" {
      # "\"Build Decay Fit Parameter Map\""
      n7 = Unbundle By Name(w42) -> ("Decay Fit Map Ctrl Refnums"=w39:T15)
      n8 = Variant To Data(Variant=w34) -> (data=w35:T32, error out=w33:errorcluster)  [unwired: 2 in]
      n9 = call "Show Animated Busy Icon with Message.vi"("Message"=w32, "Error In"=w33, "Target VI Refnum"=w40) -> ("Error Out"=w41:errorcluster)  [unwired: 8 in]
      n10 = call "AlliGator Build Decay Fit Parameter Map.vi"("error in (no error)"=w41, "Decay Fit Parameter Map Update Event Data"=w35, "Decay Fit Map Ctrl Refums"=w39, "AlliGator Internal Variables DVR"=w38) -> ("error out"=w48:errorcluster, "AlliGator Internal Variables DVR"=w37:refnum<data-value>)  [unwired: 2 in, 4 out]
      n11 = call "Hide Animated Busy Icon with Message.vi"("Error In"=w48, "Target VI reference"=w40) -> ("Error Out"=w36:errorcluster)  [unwired: 9 in]
      n12 = Bundle By Name(cluster=T6 {"AlliGator Q Event"=enum."Decay Fit Parameter Map:Change Decay Fit Parameter Map Color Palette", "Data"=variant} ("Alligator Atomic Action"), "Data"="Refresh Image") -> (w44:T6)
      n13 = call-poly "AlliGator Add Action(s) to Stack.vi"("Elements Order in Action Stack (Default: 2 BEFORE 1)"=Alligator_Elements_Order_in_Action_Stack."Enqueue 2 BEFORE 1", "Error In"=w36, "Alligator Atomic Action"=w44, "Alligator Queue Element 1"=w50) -> ("Error Out"=w43:errorcluster, "Alligator Queue Element 1 (+ 2)"=w49:T6[])  [unwired: 6 in]
    }
    frame "Decay Fit Parameter Map:Change Decay Fit Parameter Map Color Palette" {
      w57 = AlliGator_Variables_List."Decay Fit Parameter Map:Palette List" ("Alligator Variable")
      # "\"Change Decay Fit Parameter Map Color Palette\""
      n14 = call "Alligator Variables Storage.vi"("Get(F)/Set"=FALSE, "AlliGator Variable"=w57) -> ("Error Out"=w56:errorcluster, "Data out"=w60:variant)  [unwired: 7 in, 1 out]
      n15 = call-poly "Variant to Data.vi"("Variant"=w60) -> ("String Array"=w58:string[])  [unwired: 8 in]
      n16 = call-poly "Variant to Data.vi"("Variant"=w71) -> ("String"=w69:string)  [unwired: 8 in]
      n17 = call "Show Animated Busy Icon with Message.vi"("Already active? (F)"=w51, "Message"=w54, "Error In"=w56, "Target VI Refnum"=w52) -> ("Error Out"=w55:errorcluster)  [unwired: 7 in]
      n18 = Unbundle By Name(w66) -> ("Decay Fit Map Ctrl Refnums"=w65:T15)
      n19 = case shown="Default" w69 {
        selector: w69 -> [_ w98 _]
        tunnel: w70 -> [_ _ _]
        tunnel: [w77 w82 w112] -> w68
        tunnel: [w76 w90 w110] -> w64
        tunnel: ["Palette List Edited" ("Append to Message") w89 _] -> w61
        tunnel: w58 -> [w73 w86 _]
        tunnel: w57 -> [w72 w81 _]
        tunnel: w55 -> [_ _ w108]
        frame "Edit Palette List..." {
          n20 = call "Edit Image Palette List Dialog.vi"("Palette List (in)"=w73) -> ("Palette List (out)"=w80:string[])  [unwired: 10 in]
          n21 = call "Alligator Variables Storage.vi"("Get(F)/Set"=TRUE, "AlliGator Variable"=w72, "Data in"=w80) -> ("Error Out"=w78:errorcluster)  [unwired: 6 in, 2 out]
          n22 = call "AlliGator Check Selected Palette.vi"("Error In"=w78, "Image"=AlliGator_Image_Display_Type."Decay Fit Parameter Map") -> ("Error Out"=w77:errorcluster, "Image Display Palette Information"=w76:T20)  [unwired: 8 in]
        }
        frame Default {
          n23 = call "Get User Palette Choice.vi"("Palette"=w98) -> ("Error Out"=w94:errorcluster, "Palette Colors"=w96:u32[], "Palette Type"=w97:T21, "Palette Name (# Colors)"=w84:string, "Interpolate?"=w92:bool, "Built-in Palette?"=w85:bool)  [unwired: 3 in, 2 out]
          n24 = Format Into String(format string="%s", initial string="Palette selected: ", w84) -> (resulting string=w89:string)  [unwired: 1 in, 1 out]
          n25 = Bundle(cluster=T20 {"Palette Name [# Colors,int?,inv?]"="", "Palette Type"=0, "Palette Colors"=[], "Interpolate?"=FALSE} ("Image Display Palette Information"), "Palette Name [# Colors,int?,inv?]"=w84, "Palette Type"=w97, "Palette Colors"=w96, "Interpolate?"=w92) -> (w90:T20)
          n26 = call "Alligator Variables Storage.vi"("Get(F)/Set"=TRUE, "AlliGator Variable"=AlliGator_Variables_List."Decay Fit Parameter Map:Palette Information" ("Alligator Variable"), "Error In"=w94, "Data in"=w90) -> ("Error Out"=w83:errorcluster)  [unwired: 5 in, 2 out]
          n27 = case shown="False" w85 {
            tunnel: w83 -> [w106 w107]
            tunnel: [w105 w107] -> w82
            tunnel: w84 -> [w104 _]
            tunnel: w86 -> [w103 _]
            tunnel: w81 -> [w99 _]
            frame False {
              n28 = Build Array (concatenate)(w103, w104) -> (w102:string[])
              n29 = call "Remove Duplicates From 1D Array.vim"("array"=w102) -> ("array with duplicates removed"=w101:string[])  [unwired: 10 in]
              n30 = call "Alligator Variables Storage.vi"("Get(F)/Set"=TRUE, "AlliGator Variable"=w99, "Error In"=w106, "Data in"=w101) -> ("Error Out"=w105:errorcluster)  [unwired: 5 in, 2 out]
            }
            frame True {
            }
          }
        }
        frame "Refresh Image" {
          n31 = call "Alligator Variables Storage.vi"("Get(F)/Set"=FALSE, "AlliGator Variable"=AlliGator_Variables_List."Decay Fit Parameter Map:Palette Information" ("Alligator Variable"), "Error In"=w108) -> ("Error Out"=w113:errorcluster, "Data out"=w114:variant)  [unwired: 6 in, 1 out]
          n32 = Variant To Data(error in=w113, type=T20 {"Palette Name [# Colors,int?,inv?]"="", "Palette Type"=0, "Palette Colors"=[], "Interpolate?"=FALSE} ("Image Display Palette Information"), Variant=w114) -> (data=w110:T20, error out=w112:errorcluster)
        }
      }
      n33 = call "AlliGator Update Decay Fit Parameter Map Palette.vi"("error in (no error)"=w68, "Decay Fit Parameter Map Display Palette Information"=w64, "Decay Fit Map Ctrl Refums"=w65) -> ("error out"=w62:errorcluster)  [unwired: 8 in]
      n34 = call "Hide Animated Busy Icon with Message.vi"("Already active? (F)"=w51, "Error In"=w62, "Target VI reference"=w52) -> ("Error Out"=w53:errorcluster)  [unwired: 8 in]
    }
    frame "Decay Fit Parameter Map:Export All Decay Fit Parameter Maps Data as ASCII" {
      # "\"Export All Decay Fit Parameter Maps Data as ASCII\""
      n35 = call "Show Animated Busy Icon with Message.vi"("Already active? (F)"=w117, "Message"=w123, "Target VI Refnum"=w122) -> ("Error Out"=w118:errorcluster)  [unwired: 8 in]
      n36 = call "AlliGator Save All Decay Fit Parameter Maps to ASCII.vi"("error in (no error)"=w118, "Data Value Reference in"=w120) -> ("error out"=w119:errorcluster, "Data Value Reference out"=w121:refnum<data-value>, "Message"=w116:string)  [unwired: 7 in]
      n37 = call "Hide Animated Busy Icon with Message.vi"("Already active? (F)"=w117, "Error In"=w119, "Target VI reference"=w122) -> ("Error Out"=w124:errorcluster)  [unwired: 8 in]
    }
    frame "Decay Fit Parameter Map:Export Decay Fit Parameter Map Data as ASCII" {
      # "\"Export Decay Fit Parameter Map Data as ASCII\""
      n38 = call-poly "Variant to Data.vi"("Variant"=w140) -> ("Value"=w139:bool)  [unwired: 8 in]
      n39 = Unbundle By Name(w135) -> ("Decay Fit Map Ctrl Refnums.Decay Fit Parameter"=w136:refnum<vi>)
      n40 = property class="Enum (strict)"(reference=w136) -> (error out=w126:errorcluster, "Value"=w134:T34)  [unwired: 1 in, 1 out]
      n41 = call "Show Animated Busy Icon with Message.vi"("Already active? (F)"=w128, "Message"=w137, "Error In"=w126, "Target VI Refnum"=w133) -> ("Error Out"=w130:errorcluster)  [unwired: 7 in]
      n42 = call "AlliGator Save Decay Fit Parameter Map to ASCII.vi"("Fit Parameter"=w134, "error in (no error)"=w130, "Dialog?"=w139, "Data Value Reference in"=w131) -> ("error out"=w129:errorcluster, "Data Value Reference out"=w132:refnum<data-value>, "Message"=w127:string)  [unwired: 5 in]
      n43 = call "Hide Animated Busy Icon with Message.vi"("Already active? (F)"=w128, "Error In"=w129, "Target VI reference"=w133) -> ("Error Out"=w138:errorcluster)  [unwired: 8 in]
    }
    frame "Decay Fit Parameter Map:Save Decay Fit Parameter Map Image" {
      # "\"Save Decay Fit Parameter Map Image\""
      n44 = Unbundle By Name(w156) -> ("Registered Events Ctrl Refnums.Decay Fit Parameter Map Display"=w149:refnum<vi>, "Decay Fit Map Ctrl Refnums.Decay Fit Parameter"=w155:refnum<vi>)
      n45 = call-poly "Variant to Data.vi"("Variant"=w157) -> ("Value"=w148:bool)  [unwired: 8 in]
      n46 = property class="Enum (strict)"(reference=w155) -> (error out=w147:errorcluster, "Value"=w150:T34)  [unwired: 1 in, 1 out]
      n47 = call "Show Animated Busy Icon with Message.vi"("Already active? (F)"=w142, "Message"=w145, "Error In"=w147, "Target VI Refnum"=w143) -> ("Error Out"=w146:errorcluster)  [unwired: 7 in]
      n48 = call "AlliGator Save Decay Fit Parameter Map Image.vi"("Dialog?"=w148, "error in (no error)"=w146, "Fit Parameter"=w150, "Image Control Refnum"=w149, "IV DVR"=w154) -> ("error out"=w151:errorcluster, "Message"=w152:string, "IV DVR"=w153:refnum<data-value>)  [unwired: 4 in]
      n49 = call "Hide Animated Busy Icon with Message.vi"("Already active? (F)"=w142, "Error In"=w151, "Target VI reference"=w143) -> ("Error Out"=w144:errorcluster)  [unwired: 8 in]
    }
    frame "Decay Fit Parameter Map:Save-Load IRFs & Fit Data" {
      # "\"Save-Load IRFs & Fit Data\""
      n50 = Variant To Data(type=T22 {"Load/Save"=FALSE, "File Path"=path ""} ("Calibration File Information"), Variant=w171) -> (data=w169:T22, error out=w159:errorcluster)  [unwired: 1 in]
      n51 = Unbundle By Name(w169) -> ("File Path"=w168:path, "Load/Save"=w167:bool)
      n52 = call "Show Animated Busy Icon with Message.vi"("Already active? (F)"=w161, "Message"=w172, "Error In"=w159, "Target VI Refnum"=w166) -> ("Error Out"=w163:errorcluster)  [unwired: 7 in]
      n53 = call "AlliGator Save-Load IRFs & Fit Data (Map).vi"("error in (no error)"=w163, "Write(T)/Load (F)"=w167, "File Path"=w168, "Data Value Reference in"=w164) -> ("error out"=w162:errorcluster, "Data Value Reference out"=w165:refnum<data-value>, "Message"=w160:string)  [unwired: 5 in]
      n54 = call "Hide Animated Busy Icon with Message.vi"("Already active? (F)"=w161, "Error In"=w162, "Target VI reference"=w166) -> ("Error Out"=w173:errorcluster)  [unwired: 8 in]
    }
    frame "Decay Fit Parameter Map:Selected Parameter Scatterplot" {
      # "Selected Parameter Scatterplot"
      n55 = call-poly "Variant to Data.vi"("Variant"=w192) -> ("Value"=w191:i32)  [unwired: 8 in]
      n56 = Unbundle By Name(w193) -> ("Registered Events Ctrl Refnums.Lifetime Graph"=w194:refnum<vi>, "Decay Fit Map Ctrl Refnums.Decay Fit Parameter"=w189:refnum<vi>)
      n57 = property class="Enum (strict)"(reference=w189) -> (error out=w183:errorcluster, "Value"=w188:T34)  [unwired: 1 in, 1 out]
      n58 = call "Show Animated Busy Icon with Message.vi"("Already active? (F)"=w185, "Message"=w195, "Error In"=w183, "Target VI Refnum"=w190) -> ("Error Out"=w182:errorcluster)  [unwired: 7 in]
      n59 = call "AlliGator Apply Fit Result Constraints.vi"("error in (no error)"=w182, "AlliGator IV DVR in"=w181) -> ("error out"=w180:errorcluster, "Message"=w177:string, "AlliGator IV DVR out"=w179:refnum<data-value>)  [unwired: 7 in]
      n60 = call "AlliGator Plot Fit Parameter Scatterplot.vi"("Fit Parameter"=w188, "Lifetime Graph refnum"=w194, "error in (no error)"=w180, "ROI idx (2147483647: all ROIs)"=w191, "Data Value Reference in"=w179) -> ("error out"=w186:errorcluster, "Data Value Reference out"=w187:refnum<data-value>, "Message"=w184:string)  [unwired: 4 in]
      n61 = Concatenate Strings(w177, "\r\n", w184) -> (w178:string)
      n62 = call "Hide Animated Busy Icon with Message.vi"("Already active? (F)"=w185, "Error In"=w186, "Target VI reference"=w190) -> ("Error Out"=w196:errorcluster)  [unwired: 8 in]
    }
    frame "Decay Fit Parameter Map:Selected Parameter vs Intensity Scatterplot" {
      # "Selected Parameter vs Intensity"
      n63 = call-poly "Variant to Data.vi"("Variant"=w215) -> ("Value"=w214:i32)  [unwired: 8 in]
      n64 = Unbundle By Name(w216) -> ("Registered Events Ctrl Refnums.Lifetime Graph"=w217:refnum<vi>, "Decay Fit Map Ctrl Refnums.Decay Fit Parameter"=w212:refnum<vi>)
      n65 = property class="Enum (strict)"(reference=w212) -> (error out=w206:errorcluster, "Value"=w211:T34)  [unwired: 1 in, 1 out]
      n66 = call "Show Animated Busy Icon with Message.vi"("Already active? (F)"=w208, "Message"=w218, "Error In"=w206, "Target VI Refnum"=w213) -> ("Error Out"=w203:errorcluster)  [unwired: 7 in]
      n67 = call "AlliGator Apply Fit Result Constraints.vi"("error in (no error)"=w203, "AlliGator IV DVR in"=w205) -> ("error out"=w202:errorcluster, "Message"=w200:string, "AlliGator IV DVR out"=w204:refnum<data-value>)  [unwired: 7 in]
      n68 = call "AlliGator Plot Decay Fit Parameter vs Intensity Scatterplot v2.vi"("Fit Parameter"=w211, "Lifetime Graph refnum"=w217, "error in (no error)"=w202, "ROI idx (2147483647: all ROIs)"=w214, "Data Value Reference in"=w204) -> ("error out"=w209:errorcluster, "Data Value Reference out"=w210:refnum<data-value>, "Message"=w207:string)  [unwired: 4 in]
      n69 = Concatenate Strings(w200, "\r\n", w207) -> (w201:string)
      n70 = call "Hide Animated Busy Icon with Message.vi"("Already active? (F)"=w208, "Error In"=w209, "Target VI reference"=w213) -> ("Error Out"=w219:errorcluster)  [unwired: 8 in]
    }
    frame "Decay Fit Parameter Map:Parameter 2 vs Parameter 1 Scatterplot" {
      # "Parameter 2 vs Parameter 1 Scatterplot"
      n71 = Unbundle By Name(w240) -> ("Registered Events Ctrl Refnums.Lifetime Graph"=w241:refnum<vi>)
      n72 = call "Show Animated Busy Icon with Message.vi"("Already active? (F)"=w236, "Message"=w242, "Target VI Refnum"=w239) -> ("Error Out"=w234:errorcluster)  [unwired: 8 in]
      n73 = Variant To Data(error in=w234, type=T25 {"Fit Parameter 1"=enum."Offset", "Fit Parameter 2"=enum."Offset"}, Variant=w235) -> (data=w232:T25, error out=w228:errorcluster)
      n74 = Unbundle By Name(w232) -> ("Fit Parameter 1"=w231:T24, "Fit Parameter 2"=w230:T24)
      n75 = call "AlliGator Apply Fit Result Constraints.vi"("error in (no error)"=w228, "AlliGator IV DVR in"=w226) -> ("error out"=w227:errorcluster, "Message"=w223:string, "AlliGator IV DVR out"=w225:refnum<data-value>)  [unwired: 7 in]
      n76 = call "AlliGator Plot Fit Parameter 2 vs Parameter 1.vi"("Lifetime Graph refnum"=w241, "error in (no error)"=w227, "Fit Parameter 2"=w230, "Fit Parameter 1"=w231, "Data Value Reference in"=w225) -> ("error out"=w237:errorcluster, "Data Value Reference out"=w238:refnum<data-value>, "Message"=w229:string)  [unwired: 4 in]
      n77 = Concatenate Strings(w223, "\r\n", w229) -> (w224:string)
      n78 = call "Hide Animated Busy Icon with Message.vi"("Already active? (F)"=w236, "Error In"=w237, "Target VI reference"=w239) -> ("Error Out"=w243:errorcluster)  [unwired: 8 in]
    }
    frame "Decay Fit Parameter Map:Set Decay Fit Parameter Map Selection" {
      # "used in script"
      # "\"Decay Fit  Parameter Map:Set Decay Fit  Parameter Map Selection\""
      n79 = Unbundle By Name(w253) -> ("Decay Fit Map Ctrl Refnums.Decay Fit Parameter"=w252:refnum<vi>)
      n80 = Variant To Data(type=Decay_Fit_Parameters_&_Derived_Quantities_List_v2."Offset" ("Fit Parameter"), Variant=w256) -> (data=w251:T24, error out=w250:errorcluster)  [unwired: 1 in]
      n81 = property class="Enum (strict)"(reference=w252, error in=w250, "Value"=w251) -> (error out=w249:errorcluster)  [unwired: 1 out]
      n82 = Format Into String(format string="Decay Fit Parameter Map Selection set to %s", error in=w249, w251) -> (resulting string=w247:string, error out=w246:errorcluster)  [unwired: 1 in]
    }
    frame "Decay Fit Parameter Map:Update Local Decay Plots" {
      # "\"Update Local Decay Plots\""
      n83 = Variant To Data(Variant=w268) -> (data=w267:T35, error out=w264:errorcluster)  [unwired: 2 in]
      n84 = call "Show Animated Busy Icon with Message.vi"("Already active? (F)"=w259, "Message"=w258, "Error In"=w264, "Target VI Refnum"=w260) -> ("Error Out"=w262:errorcluster)  [unwired: 7 in]
      n85 = call "AlliGator Send Local Decay Plots.vi"("error in (no error)"=w262, "ROI Descriptor"=w267, "AlliGator IV DVR in"=w266) -> ("error out"=w263:errorcluster, "AlliGator IV DVR out"=w265:refnum<data-value>)  [unwired: 7 in]
      n86 = call "Hide Animated Busy Icon with Message.vi"("Already active? (F)"=w259, "Error In"=w263, "Target VI reference"=w260) -> ("Error Out"=w261:errorcluster)  [unwired: 8 in]
    }
    frame "Decay Fit Parameter Map:Python Function Decay Fit Parameters Map Event" {
      # "\"Decay Fit Parameters:Python Function Decay Fit Parameters Map Event\""
      n87 = One Button Dialog(message="Not yet supported....") -> ()  [unwired: 1 in, 1 out]
      n88 = call "Play Error Sound.vi"() -> ()  [unwired: 27 in, 1 out]
    }
    frame "Decay Fit Parameter Map:Overlay Decay Fit Parameter Map in Source Image" {
      # "\"Overlay Decay Fit Parameter Map in Source Image\""
      n89 = Unbundle By Name(w281) -> ("Decay Fit Map Ctrl Refnums.Decay Fit Parameter Map Color Scale"=w291:refnum<vi>, "Dataset Control Refnums.Image Color Scale"=w292:refnum<vi>, "Registered Events Ctrl Refnums.Source Image Display"=w290:refnum<vi>)
      n90 = Unbundle By Name(w281) -> ("Dataset Control Refnums.Save Image"=w289:refnum<vi>)
      n91 = property class="Bool (strict)"(reference=w289) -> (error out=w277:errorcluster, "Value"=w288:bool)  [unwired: 1 in, 1 out]
      n92 = call "Show Animated Busy Icon with Message.vi"("Already active? (F)"=w279, "Message"=w278, "Error In"=w277, "Target VI Refnum"=w280) -> ("Error Out"=w287:errorcluster)  [unwired: 7 in]
      n93 = call "AlliGator Overlay Decay Fit Parameter Map in Original Image.vi"("Decay Fit Parameter Map Color Scale Refnum"=w291, "Image Color Scale Refnum"=w292, "Error In"=w287, "Destination Image Control Refnum"=w290, "AlliGator IV DVR in"=w285) -> ("Error Out"=w286:errorcluster, "AlliGator IV DVR out"=w284:refnum<data-value>)  [unwired: 4 in, 1 out]
      n94 = call "Hide Animated Busy Icon with Message.vi"("Already active? (F)"=w279, "Error In"=w286, "Target VI reference"=w280) -> ("Error Out"=w276:errorcluster)  [unwired: 8 in]
      n95 = case shown="False" w288 {
        tunnel: w283 -> [w294 w300]
        tunnel: [w294 w297] -> w282
        tunnel: w276 -> [w293 w296]
        tunnel: [w293 w295] -> w275
        frame False {
        }
        frame True {
          n96 = call-poly "AlliGator Add Action(s) to Stack.vi"("Elements Order in Action Stack (Default: 2 BEFORE 1)"=Alligator_Elements_Order_in_Action_Stack."Enqueue 2 BEFORE 1", "Error In"=w296, "Alligator Atomic Action"=T6 {"AlliGator Q Event"=enum."Image:Save Displayed Image with Overlay", "Data"=variant}, "Alligator Queue Element 1"=w300) -> ("Error Out"=w295:errorcluster, "Alligator Queue Element 1 (+ 2)"=w297:T6[])  [unwired: 6 in]
        }
      }
    }
    frame "Decay Fit Parameter Map:Mouse Up" {
      # "\"Decay Fit Parameter Map:Mouse Up\""
      n97 = Variant To Data(type=T26 {"Current ROI Tool"=8, "ROI Descriptor"={"Global Rectangle"=[], "Contours"=[]}, "Shift"=FALSE, "Alt"=FALSE, "Image Display Refnum"=refnum} ("Phasor Plot Mouse Up Event Data"), Variant=w304) -> (data=w303:T26, error out=w302:errorcluster)  [unwired: 1 in]
      n98 = call "AlliGator Decay Parameters Map Mouse Up Event.vi"("error in (no error)"=w302, "Image Mouse Up Event Data"=w303, "AlliGator Actions in"=w307) -> ("error out"=w305:errorcluster, "AlliGator Actions out"=w306:T6[])  [unwired: 7 in]
    }
    frame "Decay Fit Parameter Map:Mouse Move" {
      # "\"Decay Fit Parameter Map:Mouse Move\""
      n99 = Unbundle By Name(w315) -> ("Decay Fit Map Ctrl Refnums"=w310:T15)
      n100 = call "AlliGator Display Current Decay Fit Parameter Map (X,Y, I).vi"("Decay Fit Map Ctrl Refums"=w310, "error in (no error)"=w313, "AlliGator Internal Variables DVR"=w312) -> ("error out"=w314:errorcluster, "AlliGator Internal Variables DVR"=w311:refnum<data-value>)  [unwired: 7 in]
    }
    frame "Decay Fit Parameter Map:Display Range Mouse Move" {
      # "\"Decay Fit Parameter Map:Display Range Mouse Move\""
      n101 = Unbundle By Name(w319) -> ("Decay Fit Map Ctrl Refnums.Decay Fit Parameter Map Display Range"=w318:refnum<vi>)
      n102 = call "Extend Display Range to Match Slider(s).vi"("error in (no error)"=w321, "Display Range"=w318) -> ("error out"=w320:errorcluster)  [unwired: 7 in, 2 out]
      n103 = Variant To Data(error in=w320, Variant=w324) -> (data=w322:T24, error out=w323:errorcluster)  [unwired: 1 in]
      n104 = call "AlliGator Decay Parameter Range Mouse Move Event.vi"("Error In"=w323, "Decay Fit Parameter"=w322, "AlliGator Actions in"=w327) -> ("Error Out"=w325:errorcluster, "AlliGator Actions out"=w326:T6[])  [unwired: 7 in]
    }
    frame "Decay Fit Parameter Map:Change Map Resolution" {
      w334 = TRUE ("Get(F)/Set")
      w349 = TRUE  # Parameter changed
      w333 = AlliGator_Variables_List."Decay Fit Parameter Map:Y Resolution" ("Alligator Variable")
      w337 = AlliGator_Variables_List."Decay Fit Parameter Map:X Resolution" ("Alligator Variable")
      n105 = call "Alligator Variables Storage.vi"("AlliGator Variable"=w337, "Error In"=w354) -> ("Error Out"=w355:errorcluster, "Data out"=w359:variant)  [unwired: 7 in, 1 out]
      n106 = Unbundle By Name(w345) -> ("Decay Fit Map Ctrl Refnums.Decay Fit Parameter"=w344:refnum<vi>)
      n107 = call-poly "Variant to Data.vi"("Variant"=w359) -> ("Value"=w358:i32)  [unwired: 8 in]
      n108 = call "Alligator Variables Storage.vi"("AlliGator Variable"=w333, "Error In"=w355) -> ("Error Out"=w356:errorcluster, "Data out"=w360:variant)  [unwired: 7 in, 1 out]
      n109 = call-poly "Variant to Data.vi"("Variant"=w360) -> ("Value"=w357:i32)  [unwired: 8 in]
      n110 = property class="Enum (strict)"(reference=w344) -> ("Value"=w343:T24)  [unwired: 1 in, 2 out]
      n111 = call "AlliGator Decay Fit Parameter Map Size Dialog.vi"("error in (no error)"=w356, "Y Resolution"=w357, "X Resolution"=w358, "Message"="Enter the original dataset's X and Y resolution:") -> ("error out"=w338:errorcluster, "Y Resolution"=w331:i32, "X Resolution"=w336:i32)  [unwired: 4 in, 1 out]
      n112 = Bundle(cluster=T32 {"Parameter"=enum."Offset", "Parameter changed"=FALSE} ("output cluster"), "Parameter"=w343, "Parameter changed"=w349) -> (w347:T32)
      n113 = call "Alligator Variables Storage.vi"("Get(F)/Set"=w334, "AlliGator Variable"=w337, "Error In"=w338, "Data in"=w336) -> ("Error Out"=w335:errorcluster)  [unwired: 5 in, 2 out]
      n114 = Bundle By Name(cluster=T6 {"AlliGator Q Event"=enum."Decay Fit Parameter Map:Build Decay Fit Parameter Map", "Data"=variant} ("Alligator Atomic Action"), "Data"=w347) -> (w348:T6)
      n115 = call "Alligator Variables Storage.vi"("Get(F)/Set"=w334, "AlliGator Variable"=w333, "Error In"=w335, "Data in"=w331) -> ("Error Out"=w332:errorcluster)  [unwired: 5 in, 2 out]
      n116 = call-poly "AlliGator Add Action(s) to Stack.vi"("Elements Order in Action Stack (Default: 2 BEFORE 1)"=Alligator_Elements_Order_in_Action_Stack."Enqueue 2 BEFORE 1", "Error In"=w332, "Alligator Atomic Action"=w348, "Alligator Queue Element 1"=w353) -> ("Error Out"=w342:errorcluster, "Alligator Queue Element 1 (+ 2)"=w352:T6[])  [unwired: 6 in]
      n117 = Format Into String(format string="New Decay Fit Parameter Map Resolution:\nX Resolution: %d\nY Resolution: %d", error in=w342, w336, w331) -> (resulting string=w339:string, error out=w341:errorcluster)  [unwired: 1 in]
    }
    frame "Decay Fit Parameter Map:Variance Significance Maps" {
      n118 = call "Show Animated Busy Icon with Message.vi"("Already active? (F)"=w376, "Message"=w379, "Error In"=w386, "Target VI Refnum"=w377) -> ("Error Out"=w366:errorcluster)  [unwired: 7 in]
      n119 = call "AlliGator Enter Power Law Parameters Dialog.vi"("Error In"=w366) -> ("Error Out"=w365:errorcluster, "Power Law Parameters out"=w367:T36)  [unwired: 8 in, 1 out]
      n120 = call "AlliGator Lifetime Variance Maps Calculation.vi"("AlliGator Ctrl Refnums"=w373, "error in (no error)"=w365, "Power Law Parameters"=w367, "AlliGator IV DVR in"=w387) -> ("error out"=w375:errorcluster, "Parameter Map Update Event Data"=w370:T37, "AlliGator IV DVR out"=w369:refnum<data-value>, "Message"=w371:string)  [unwired: 4 in]
      n121 = Unbundle By Name(w373) -> ("Parameter Map Ctrl Refnums"=w372:T16)
      n122 = call "AlliGator Build Parameter Map.vi"("error in (no error)"=w375, "Parameter Map Update Event Data"=w370, "Parameter Map Ctrl Refums"=w372, "AlliGator Internal Variables DVR"=w369) -> ("error out"=w374:errorcluster, "AlliGator Internal Variables DVR"=w368:refnum<data-value>)  [unwired: 3 in, 3 out]
      n123 = Bundle By Name(cluster=T6 {"AlliGator Q Event"=enum."Parameter Map:Change Parameter Map Color Palette", "Data"=variant} ("Alligator Atomic Action"), "Data"="Refresh Image") -> (w383:T6)
      n124 = call "Hide Animated Busy Icon with Message.vi"("Already active? (F)"=w376, "Error In"=w374, "Target VI reference"=w377) -> ("Error Out"=w378:errorcluster)  [unwired: 8 in]
      n125 = call-poly "AlliGator Add Action(s) to Stack.vi"("Elements Order in Action Stack (Default: 2 BEFORE 1)"=Alligator_Elements_Order_in_Action_Stack."Enqueue 2 BEFORE 1", "Error In"=w378, "Alligator Atomic Action"=w383, "Alligator Queue Element 1"=w382) -> ("Alligator Queue Element 1 (+ 2)"=w381:T6[])  [unwired: 6 in, 1 out]
    }
    frame "Decay Fit Parameter Map:Fit Result Constraints Window" {
      n126 = call "AlliGator Get Ancillary Window Path.vi"("AlliGator Window"=AlliGator_Windows_List."Fit Result Constraints Window" ("AlliGator Windows")) -> ("Error Out"=w390:errorcluster, "VI Path"=w391:path)  [unwired: 9 in]
      n127 = call "Run Vi.vi"("VI Path"=w391, "error in (no error)"=w390, "Start Hidden? (F)"=TRUE) -> ()  [unwired: 5 in, 2 out]
    }
  }
  "Data Value Reference out" <- w17
  "error out" <- w14
  "AlliGator Q Elements out" <- w9
  "Script out" <- w6
  n128 = call "Get Current Message Text Format.vi"("Text Format"=w1) -> ("Message Formatting"=w3:T2)  [unwired: 8 in, 1 out]
  n129 = call "AlliGator Package Notebook Messages.vi"("Message Formatting"=w3, "Message"=w4, "AlliGator Q Event in"="AlliGator Q Event in") -> ("[Notebook Message]"=→"[Notebook Message]":T1[])  [unwired: 8 in]
